vi "PM100-PM200 Utility.vi"() -> ()   [LabVIEW 2015]
uses:
  <vilib>/ptbypt/NI_PtbyPt.lvlib
  <vilib>/Utility/config.llb/NI_LVConfig.lvlib
  <vilib>/Utility/config.llb/Read Key (I32).vi
  <vilib>/Utility/config.llb/Write Key (I32).vi
  <vilib>/Utility/config.llb/Write Key (U32).vi
  StateMachine.ctl
  <vilib>/regexp/Match Regular Expression.xnode
  <vilib>/Utility/config.llb/Write Key (Double).vi
  <vilib>/Utility/config.llb/Write Key (Boolean).vi
  <vilib>/Utility/NIReport.llb/NI_ReportGenerationCore.lvlib
  <vilib>/printing/EasyPrintingControls.llb/contents.ctl
  <vilib>/printing/EasyPrintingControls.llb/orientation.ctl
  <vilib>/printing/EasyPrintingControls.llb/panel_scaling_for_page.ctl
  <vilib>/printing/EasyPrintingControls.llb/margin_values.ctl
  <vilib>/printing/EasyPrintingControls.llb/measurement_system.ctl
  <vilib>/printing/EasyPrintingControls.llb/margins.ctl
  <vilib>/printing/EasyPrintingControls.llb/printing_method.ctl
  <vilib>/printing/EasyPrintingControls.llb/color_or_monochrome.ctl
  <vilib>/printing/EasyPrintingControls.llb/printer_options.ctl
  <vilib>/printing/EasyPrintingControls.llb/page_headers.ctl
  <vilib>/printing/EasyPrintingControls.llb/page_header_content_options.ctl
  <vilib>/printing/EasyPrintingControls.llb/page_header_options.ctl
  <vilib>/printing/EasyPrintingControls.llb/layout_options.ctl
  <vilib>/printing/EasyPrintingControls.llb/report_type.ctl
  <vilib>/Utility/config.llb/Read Key (Boolean).vi
  <vilib>/Analysis/NI_AALBase.lvlib
  <vilib>/Utility/config.llb/Read Key (Double).vi
  <vilib>/Instr/_visa.llb/VISA GPIB Control REN Mode.ctl
  <vilib>/printing/EasyPrinting.llb/Easy Print VI Panel or Documentation (path).vi
panel:
  in  "att":string
  in  "Print":bool
  in  "LTM":bool caption="Long Term Measurement"
  out "Log":bool
  in  "Arm":string
  out "VI_Path":path
  in  "Button9":bool
  in  "Button10":bool
  out "Adapter":i16
  in  "Flag1":string
  in  "Flag0":string
  out "Tau":dbl
  out "Tau?":bool
  out "Temp":bool
  out "ARM":bool
  out "Stop":bool
  in  "Frame":T1
  out "Sensor?":bool
  out "SensType":i32(ring) items=["No Sensor", "Photo", "Thermo", "Pyro"]
  out "AUTO?":bool
  out "DiaIni":dbl
  out "PM100D":refnum<visa-resource-name>
  in  "Type":u16
  in  "BW":u16(ring) items=["HIGH", "LOW"]
  in  "ACC":string(combo)
  in  "Trig":dbl=5.0
  out "AOutcm²":dbl=5.0
  in  "LambdaMax":dbl=1100.0
  in  "LambdaMin":dbl=400.0
  in  "Lambda":dbl=635.0
  in  "Range Array":string[](array[string])=["AUTO", "50nA", "500nA", "5uA", "50uA", "500uA", "5mA"]
  out "Dia":dbl
  out "SlideMulti":dbl
  in  "AVG":u32=100
  out "FileRefnum":refnum<file>
  in  "File?":bool
  in  "Samples":u32=100
  out "N":u32
  out "Data":dbl
  in  "Interval":dbl=500.0
  in  "MainUnits":enum16{"W", "V", "J", "dBm", "A"}(ring)
  in  "Digits":i32=4
  in  "Sub2":enum16{"Off", "Max", "Ratio", "Area", "Second"}(ring)=enum."Max"
  in  "Sub1":enum16{"Off", "Min", "Freq", "Temp", "Res"}(ring)=enum."Min"
  in  "Button8":bool
  in  "Button7":bool
  in  "Button6":bool
  in  "Button4":bool
  in  "Button3":bool
  in  "Button2":bool
  in  "Button5":bool
  in  "Button1":bool
  out "Header":string
  out "Slide":u32(slide) scale=0.0..1000.0
  out "Sub1":string
  out "Sub2":string
  out "Readout":string
  out "FastOut":bool
  in  "FastIn":bool
  in  "Int.":i32=10 caption="Intervals" min=1 max=9999 step=1
  in  "LogCfg":string
  in  "Stat2":string
  in  "Stat1":string
  in  "Stat0":string
  out "Histogram":T2(graph)
  in  "LogData":string
  out "YT":cluster{timestamp[], dbl[]}(graph)
  out "Unit":string="Power / W"
  out "Chart_E":dbl(graph)
  out "Chart_P":dbl(graph)
  in  "Att":dbl format="%_6g"
  out "Wav":bool
  in  "Scale":bool
  out "H":dbl
  in  "Unt":string
  in  "LFP":path caption="Log-File Path"
  in  "Imp":bool
  out "N2":u32
  out "T":dbl
  in  "EMM":bool caption="Environmental Data"
  out "Hum":string caption="Rel. Humidity"
  out "Temp":string caption="Temperature"
  in  "Exp":bool
  in  "ClrGr":bool
  in  "XScaleFit":bool
  in  "YScaleRep":bool
  in  "YScaleFit":bool
  # "PM100 / PM200 Series\nOptical Power and Energy Meters"
  # "Instrument Setup"
  # "Count >"
  # "Histogram"
  # "Y-Scale"
  # "Scale Fit"
  # "Map Mode"
  # "X-Scale"
  # "Scale Fit"
  # "Scale"
  # "PM100 Utility\nVersion 4.91\n10-JUL-2013\nwww.thorlabs.com"
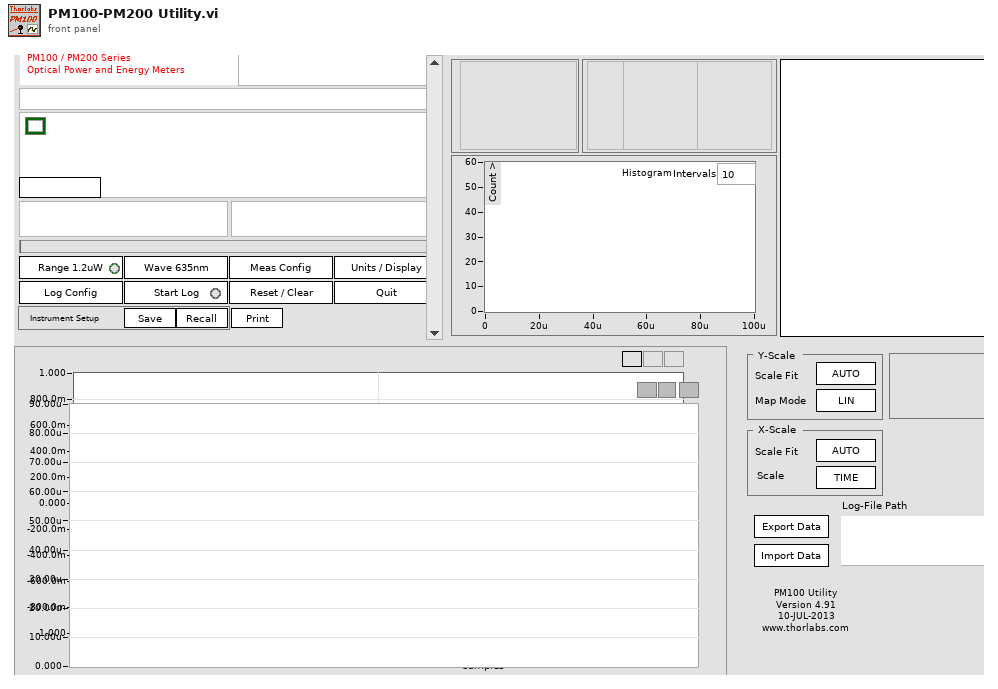
[diagram p1: front panel]
types:
  T1 = typedef "StateMachine.ctl" = enum16{"Initialize", "Load Settings", "20", "30", "40", "60", "80", "100", "120", "130", "140", "150", "160", "180", "200", "220", "240", "260", "280", "300", "320", "340", "360", "380", "400", "420", "440", "460", "480", "500", "Error", "Save Settings", "Stop"}
  T2 = cluster{"X Values":dbl[], "Histogram: h(x)":i32[]}
  T3 = enum16{"open", "replace", "create", "open or create", "replace or create", "replace or create with confirmation"}
  T4 = cluster{"X Values":i32[], "Histogram: h(x)":i32[]}
  T5 = typedef "NI_ReportGenerationCore.lvlib/layout_options.ctl" = cluster{"orientation (unchanged)":T6, "panel scaling for page (unchanged)":T7, "margins":T8, "printer options":T11, "page header options":T14}
  T6 = typedef "NI_ReportGenerationCore.lvlib/orientation.ctl" = u16
  T7 = typedef "NI_ReportGenerationCore.lvlib/panel_scaling_for_page.ctl" = u16
  T8 = typedef "NI_ReportGenerationCore.lvlib/margins.ctl" = cluster{"override VI margins (false)":bool, "margins (1.00)":T9, "measurement system (default)":T10}
  T9 = typedef "NI_ReportGenerationCore.lvlib/margin_values.ctl" = cluster{"top":dbl, "left":dbl, "right":dbl, "bottom":dbl}
  T10 = typedef "NI_ReportGenerationCore.lvlib/measurement_system.ctl" = u16
  T11 = typedef "NI_ReportGenerationCore.lvlib/printer_options.ctl" = cluster{"destination printer name (current)":string, "printing method (unchanged)":T12, "color or monochrome (unchanged)":T13}
  T12 = typedef "NI_ReportGenerationCore.lvlib/printing_method.ctl" = u16
  T13 = typedef "NI_ReportGenerationCore.lvlib/color_or_monochrome.ctl" = u16
  T14 = typedef "NI_ReportGenerationCore.lvlib/page_header_options.ctl" = cluster{"page headers (unchanged)":T15, "page header content options":T16}
  T15 = typedef "NI_ReportGenerationCore.lvlib/page_headers.ctl" = u16
  T16 = typedef "NI_ReportGenerationCore.lvlib/page_header_content_options.ctl" = cluster{"Include VI Name":bool, "Include VI Path":bool, "Include Last Modification Date":bool, "Include Date Printed":bool, "Include Page Number":bool, "Include VI Icon":bool}
  T17 = typedef "NI_LVConfig.lvlib/Config Data RefNum.ctl" = refnum<k1>
  T18 = typedef "NI_ReportGenerationCore.lvlib/report_type.ctl" = u16
  T19 = typedef "NI_ReportGenerationCore.lvlib/contents.ctl" = u16
  T20 = enum32{"invalid app kind", "Development System", "Run Time System", "Student Edition", "Embedded LabVIEW", "Evaluation", "Custom"}
  T21 = typedef "VISA GPIB Control REN Mode.ctl" = u16
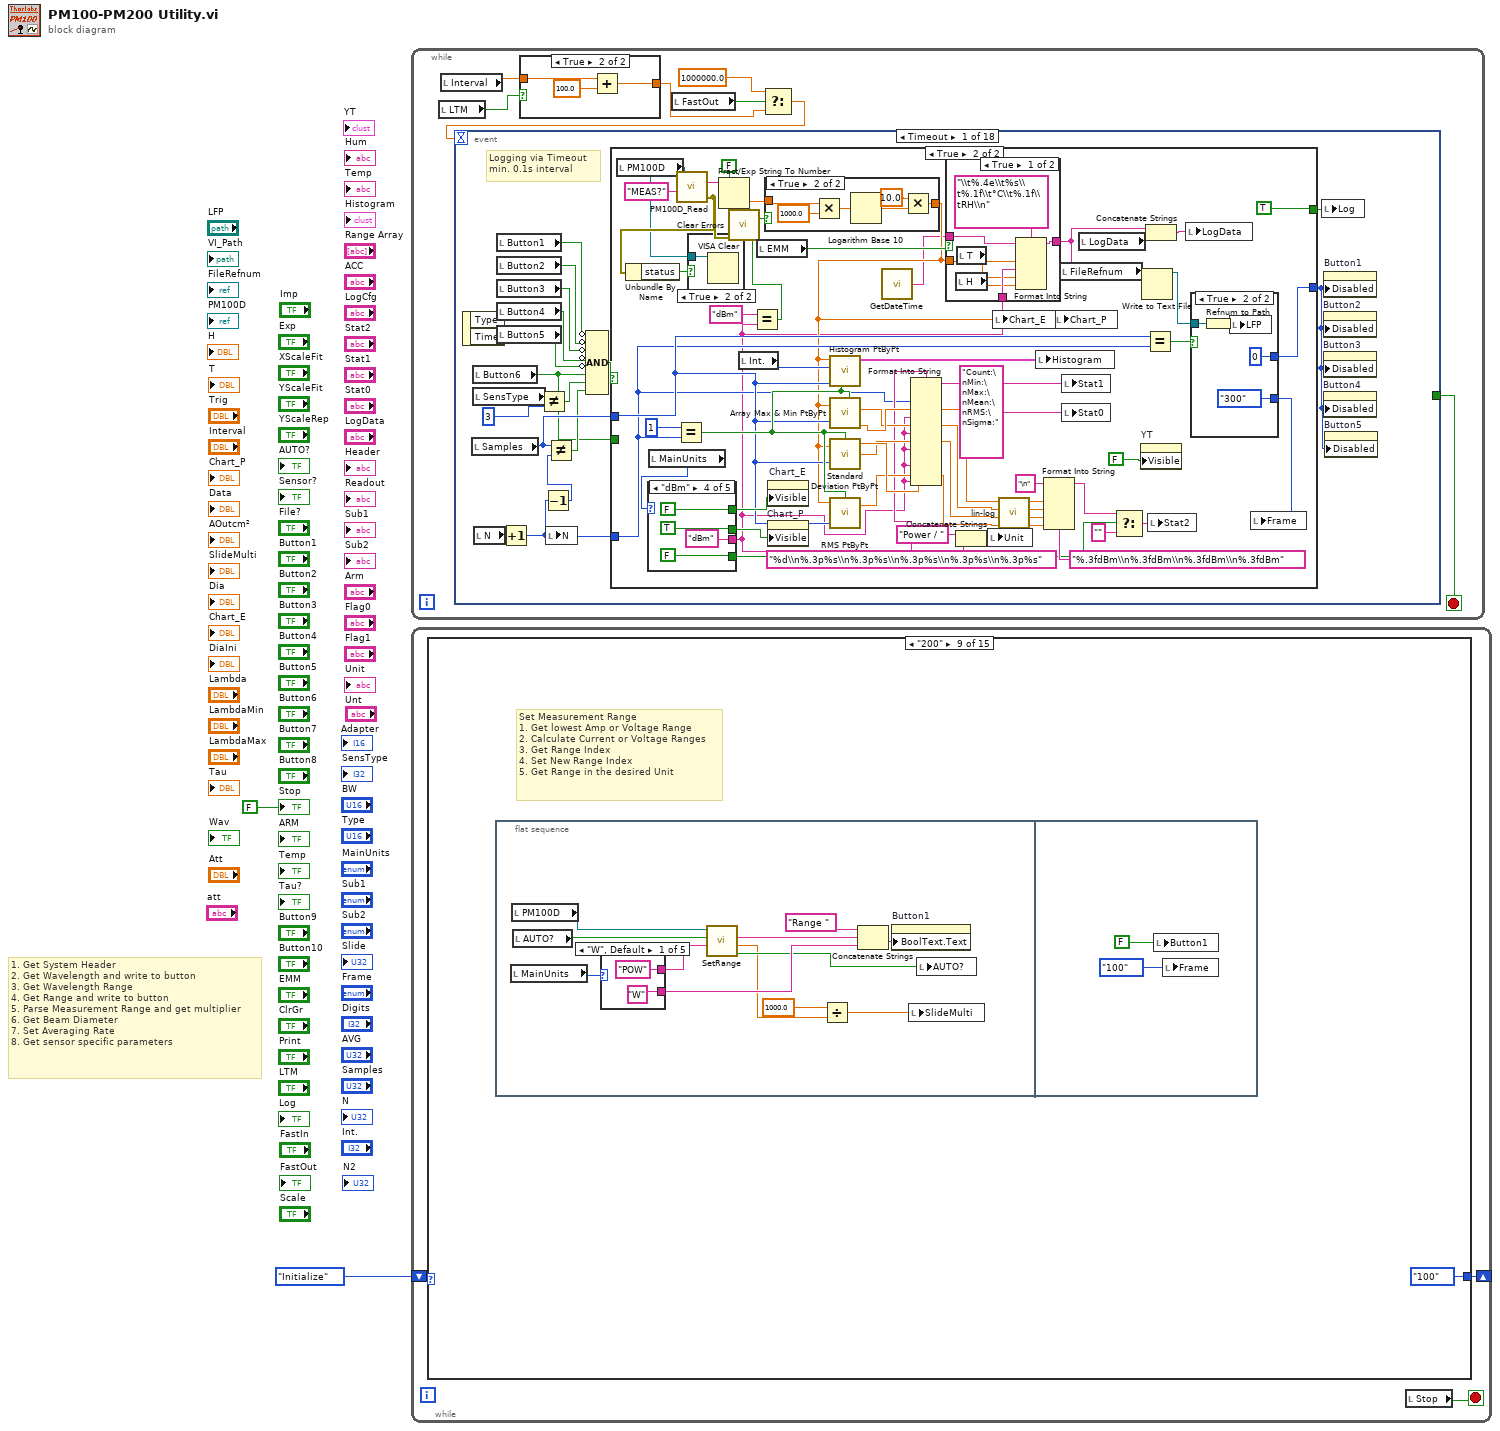
[diagram p0: block diagram]
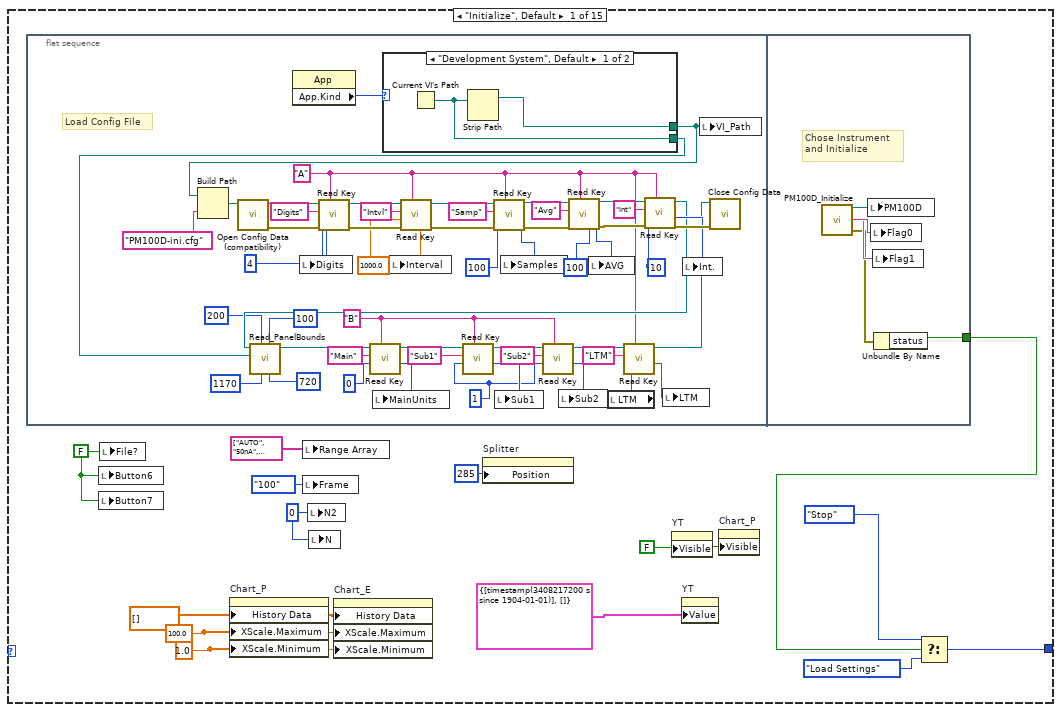
[diagram p2: hidden frame]
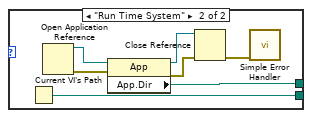
[diagram p3: hidden frame]
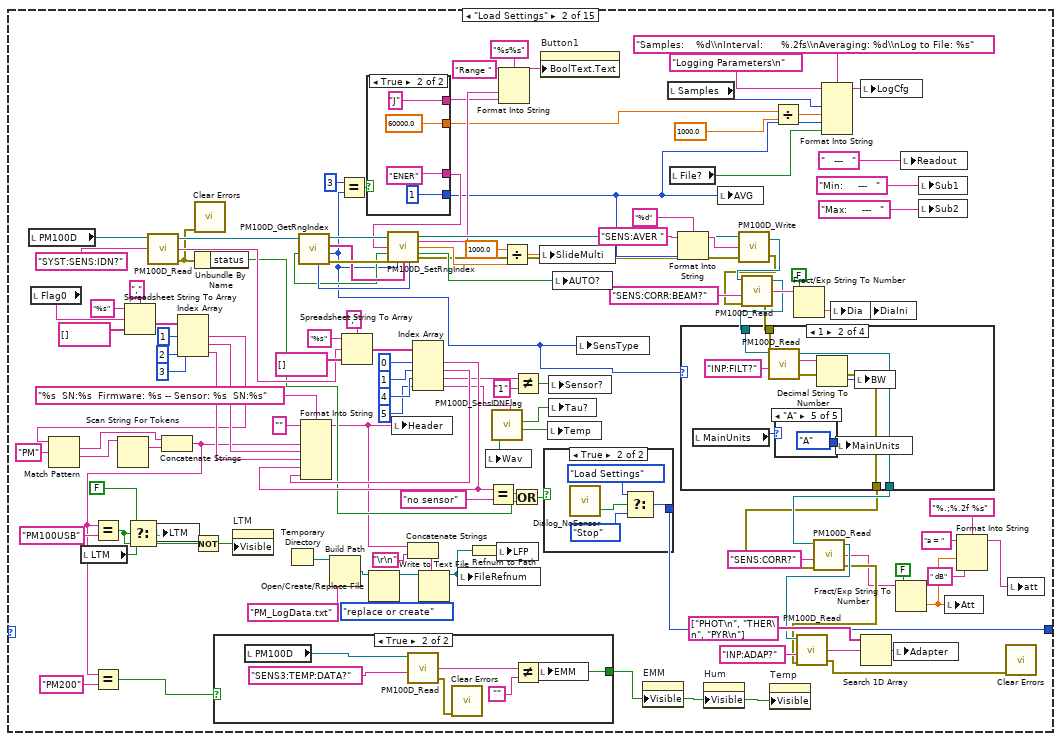
[diagram p4: hidden frame]
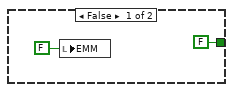
[diagram p5: hidden frame]
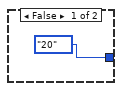
[diagram p6: hidden frame]
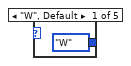
[diagram p8: hidden frame]
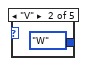
[diagram p9: hidden frame]
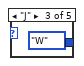
[diagram p10: hidden frame]
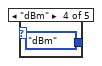
[diagram p11: hidden frame]
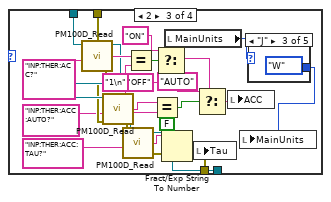
[diagram p12: hidden frame]
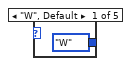
[diagram p13: hidden frame]
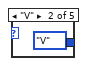
[diagram p14: hidden frame]
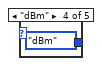
[diagram p15: hidden frame]
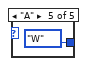
[diagram p16: hidden frame]
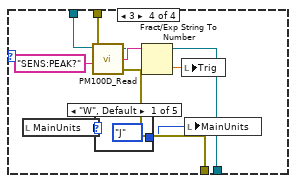
[diagram p17: hidden frame]
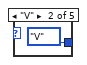
[diagram p18: hidden frame]
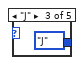
[diagram p19: hidden frame]
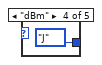
[diagram p20: hidden frame]
diagram:
  # "1. Get System Header\n2. Get Wavelength and write to button\n3. Get Wavelength Range\n4. Get Range and write to button\n5. Parse Measurement Range and get multiplier\n6. Get Beam Diameter\n7. Set Averaging Rate\n8. Get sensor specific parameters"
  n1 = while {
    stop <- w9 stop-if-true
    n2 = local read "LTM"() -> (w7:bool)
    n3 = local read "Interval"() -> (w8:dbl)
    n4 = case shown="True" w7 {
      tunnel: w8 -> [w10 w12]
      tunnel: [w10 w11] -> w4
      frame False {
      }
      frame True {
        n5 = Add(x=w12, y=100.0) -> (x+y=w11:dbl)
      }
    }
    n6 = local read "FastOut"() -> (w6:bool)
    n7 = Select(t=1000000.0, s=w6, f=w4) -> (s? t:f=w5:dbl)
    n8 = event shown="[0] Timeout" {
      selector: _ -> [_ _ _ _ _ _ _ _ _ _ _ _ _ _ _ _ _ _]
      dyn-events: _ -> [_ _ _ _ _ _ _ _ _ _ _ _ _ _ _ _ _ _]
      timeout: w5 -> [_ _ _ _ _ _ _ _ _ _ _ _ _ _ _ _ _ _]
      tunnel: [_ _ _ _ _ _ _ _ _ TRUE ("NewVal") _ _ _ _ _ _ w464 TRUE ("NewVal")] -> w9
      event Timeout {
        # "Logging via Timeout\nmin. 0.1s interval"
        n9 = event-data() -> ()  [unwired: 1 in, 2 out]
        n10 = local read "Samples"() -> (w27:u32)
        n11 = local read "Button6"() -> (w15:bool)
        n12 = local read "SensType"() -> (w25:i32)
        n13 = local read "N"() -> (w29:u32)
        n14 = local read "Button1"() -> (w16:bool)
        n15 = local read "Button2"() -> (w17:bool)
        n16 = local read "Button3"() -> (w18:bool)
        n17 = local read "Button4"() -> (w19:bool)
        n18 = local read "Button5"() -> (w20:bool)
        n19 = Increment(x=w29) -> (x+1=w26:u32)
        n20 = Not Equal?(x=w25, y=3) -> (x != y?=w22:bool)
        n21 = Decrement(x=w26) -> (x-1=w28:u32)
        n22 = Not Equal?(x=w27, y=w28) -> (x != y?=w23:bool)
        n23 = local write "N"(w26) -> ()
        n24 = Compound Arithmetic op=AND(invert w16, invert w17, invert w18, invert w19, invert w20, w15, w22, w23) -> (w30:bool)
        n25 = case shown="True" w30 {
          tunnel: w27 -> [w36 w61]
          tunnel: w26 -> [w32 w60]
          tunnel: [0 w49] -> w21
          tunnel: w15 -> [w38 _]
          tunnel: [FALSE TRUE] -> w14
          frame False {
            n26 = Equal?(x=w38, y=TRUE) -> (x = y?=w35:bool)
            n27 = Less?(x=w32, y=w36) -> (x < y?=w34:bool)
            n28 = And(x=w35, y=w34) -> (x .and. y?=w33:bool)
            n29 = case shown="True" w33 {
              frame False {
                n30 = local write "Button6"(FALSE ("Button6")) -> ()
                n31 = local write "N"(i16 0 ("N")) -> ()
              }
              frame True {
                n32 = disable-structure shown="Enabled" {
                  frame Enabled {
                    n33 = local read "N"() -> (w43:u32)
                    n34 = Decrement(x=w43) -> (x-1=w42:u32)
                    n35 = local write "N"(w42) -> ()
                  }
                  frame Disabled {
                  }
                }
              }
            }
          }
          frame True {
            n36 = local read "PM100D"() -> (w45:refnum<visa-resource-name>)
            n37 = local read "MainUnits"() -> (w90:enum16{"W", "V", "J", "dBm", "A"})
            n38 = case shown="\"dBm\"" w90 {
              tunnel: ["W" "V" "J" "dBm" "A"] -> w53
              tunnel: [w123 w126 w128 FALSE w136] -> w74
              tunnel: [FALSE w126 TRUE FALSE w136] -> w73
              tunnel: [w123 TRUE w128 TRUE TRUE] -> w72
              frame "W", Default {
                w123 = TRUE
              }
              frame "V" {
                w126 = FALSE
              }
              frame "J" {
                w128 = FALSE
              }
              frame "dBm" {
              }
              frame "A" {
                w136 = FALSE
              }
            }
            n39 = Equal?(x=i16 1, y=w60) -> (x = y?=w91:bool)
            n40 = call "PM100D_Read.vi"("Command"="MEAS?", "VISA in"=w45) -> ("error out"=w46:errorcluster, "ReadValue"=w58:string)  [unwired: 2 in, 1 out]
            n41 = Unbundle By Name(w46) -> ("status"=w44:bool)
            n42 = case shown="True" w44 {
              tunnel: w45 -> [_ w96]
              frame False {
              }
              frame True {
                n43 = VISA Clear(VISA resource name=w96) -> ()  [unwired: 1 in, 2 out]
              }
            }
            n44 = Fract/Exp String To Number(use system decimal point (T)=FALSE, string=w58) -> (number=w55:dbl)  [unwired: 2 in, 1 out]
            n45 = call <vilib>:"Clear Errors.vi"("error in (no error)"=w46) -> ()  [unwired: 5 in, 2 out]
            n46 = local read "Int."() -> (w71:i32)
            n47 = Equal?(x="dBm", y=w53) -> (x = y?=w51:bool)
            n48 = local read "EMM"() -> (w67:bool)
            n49 = case shown="True" w51 {
              tunnel: w55 -> [w97 w99]
              tunnel: [w97 w98] -> w54
              frame False {
              }
              frame True {
                n50 = Multiply(x=w99, y=1000.0) -> (x*y=w101:dbl)
                n51 = Logarithm Base 10(1:w101) -> (0:w103:dbl)
                n52 = Multiply(x=10.0, y=w103) -> (x*y=w98:dbl)
              }
            }
            n53 = property on="Chart_E" class="WFChart (strict)"("Visible"=w73) -> ()  [unwired: 2 in, 2 out]
            n54 = property on="Chart_P" class="WFChart (strict)"("Visible"=w72) -> ()  [unwired: 2 in, 2 out]
            n55 = call <vilib>:"Histogram PtByPt.vi"("initialize"=w91, "sample length"=w61, "intervals"=w71, "x"=w54) -> ("Histogram Graph"=w94:T2)  [unwired: 4 in, 3 out]
            n56 = call <vilib>:"Array Max & Min PtByPt.vi"("input data point"=w54, "sample length"=w61, "initialize"=w91) -> ("max value"=w82:dbl, "min value"=w83:dbl)  [unwired: 3 out]
            n57 = call <vilib>:"Standard Deviation PtByPt.vi"("x"=w54, "sample length"=w61, "initialize"=w91) -> ("standard deviation"=w89:dbl, "mean"=w81:dbl)  [unwired: 1 out]
            n58 = call <vilib>:"RMS PtByPt.vi"("initialize"=w91, "sample length"=w61, "x"=w54) -> ("rms value"=w80:dbl)  [unwired: 1 in, 1 out]
            n59 = call "GetDateTime.vi"() -> ("date&time"=w47:string)
            n60 = Format Into String(format string="%d\\n%.3p%s\\n%.3p%s\\n%.3p%s\\n%.3p%s\\n%.3p%s", w60, w83, w53, w82, w53, w81, w53, w80, w53, w89, w53) -> (resulting string=w93:string)  [unwired: 2 in, 1 out]
            n61 = case shown="True" w67 {
              tunnel: [w115 w120] -> w50
              tunnel: w54 -> [w114 w119]
              tunnel: w53 -> [w113 w118]
              tunnel: w47 -> [w112 w117]
              frame True {
                n62 = local read "H"() -> (w110:dbl)
                n63 = local read "T"() -> (w111:dbl)
                n64 = Format Into String(format string="\\t%.4e\\t%s\\t%.1f\\t°C\\t%.1f\\tRH\\n", initial string=w112, w114, w113, w111, w110) -> (resulting string=w115:string)  [unwired: 1 in, 1 out]
              }
              frame False {
                n65 = Format Into String(format string="\\t%.4e\\t%s\\n", initial string=w117, w119, w118) -> (resulting string=w120:string)  [unwired: 1 in, 1 out]
              }
            }
            n66 = Concatenate Strings("Power / " ("string"), w53) -> (w69:string)
            n67 = local write "Unit"(w69) -> ()
            n68 = local write "Chart_E"(w54) -> ()
            n69 = call "lin-log.vi"("W In 1"=w80, "W In 2"=w81, "W In 3"=w82, "W In 4"=w83) -> ("dBm Out 1"=w84:dbl, "dBm Out 2"=w85:dbl, "dBm Out 3"=w86:dbl, "dBm Out 4"=w87:dbl)
            n70 = local write "Histogram"(w94) -> ()
            n71 = Format Into String(format string="%.3fdBm\\n%.3fdBm\\n%.3fdBm\\n%.3fdBm", initial string="\n", w87, w86, w85, w84) -> (resulting string=w78:string)  [unwired: 1 in, 1 out]
            n72 = local write "Chart_P"(w54) -> ()
            n73 = local read "FileRefnum"() -> (w64:refnum<file>)
            n74 = local write "Stat1"(w93) -> ()
            n75 = local write "Stat0"("Count:\nMin:\nMax:\nMean:\nRMS:\nSigma:" ("Stat0")) -> ()
            n76 = local read "LogData"() -> (w65:string)
            n77 = Select(t=w78, s=w74, f="") -> (s? t:f=w77:string)
            n78 = property on="YT" class="XYGraph (strict)"("Visible"=FALSE) -> ()  [unwired: 2 in, 2 out]
            n79 = Write to Text File(file (use dialog)=w64, text=w50) -> (refnum out=w59:refnum<file>)  [unwired: 2 in, 2 out]
            n80 = Equal?(x=w61, y=w60) -> (x = y?=w62:bool)
            n81 = Concatenate Strings(w50, w65) -> (w66:string)
            n82 = local write "Stat2"(w77) -> ()
            n83 = local write "LogData"(w66) -> ()
            n84 = case shown="True" w62 {
              tunnel: [StateMachine."120" ("Frame") StateMachine."300" ("Frame")] -> w63
              tunnel: w59 -> [_ w108]
              tunnel: [2 0] -> w49
              frame False {
              }
              frame True {
                n85 = Refnum to Path(1:w108) -> (0:w107:path)
                n86 = local write "LFP"(w107) -> ()
              }
            }
            n87 = local write "Frame"(w63) -> ()
          }
        }
        n88 = local write "Log"(w14) -> ()
        n89 = property on="Button1" class="Bool (strict)"("Disabled"=w21) -> ()  [unwired: 2 in, 2 out]
        n90 = property on="Button2" class="Bool (strict)"("Disabled"=w21) -> ()  [unwired: 2 in, 2 out]
        n91 = property on="Button3" class="Bool (strict)"("Disabled"=w21) -> ()  [unwired: 2 in, 2 out]
        n92 = property on="Button4" class="Bool (strict)"("Disabled"=w21) -> ()  [unwired: 2 in, 2 out]
        n93 = property on="Button5" class="Bool (strict)"("Disabled"=w21) -> ()  [unwired: 2 in, 2 out]
      }
      event "att": Mouse Down {
        n94 = event-data() -> ()  [unwired: 1 in, 8 out]
        n95 = local write "N2"(u32 0 ("N")) -> ()
        n96 = local write "Frame"(StateMachine."240" ("Frame")) -> ()
      }
      event "Button1": Value Change {
        # "Set Range - goto Frame 200"
        n97 = event-data() -> ("NewVal"=w143:bool)  [unwired: 1 in, 5 out]
        n98 = Equal?(x=w143, y=TRUE) -> (x = y?=w141:bool)
        n99 = case shown="True" w141 {
          frame False {
          }
          frame True {
            n100 = local write "Frame"(StateMachine."200" ("Frame")) -> ()
          }
        }
        n101 = local write "N2"(u32 0 ("N2")) -> ()
      }
      event "Button2": Value Change {
        # "Set Wavelength - goto Frame 220"
        n102 = event-data() -> ("NewVal"=w148:bool)  [unwired: 1 in, 5 out]
        n103 = Equal?(x=w148, y=TRUE) -> (x = y?=w146:bool)
        n104 = case shown="True" w146 {
          frame False {
          }
          frame True {
            n105 = local write "Frame"(StateMachine."220" ("Frame")) -> ()
          }
        }
        n106 = local write "N2"(u32 0 ("N2")) -> ()
      }
      event "Button3": Value Change {
        # "Set Measuremnt Configuration - goto Frame 240"
        n107 = event-data() -> ("NewVal"=w153:bool)  [unwired: 1 in, 5 out]
        n108 = Equal?(x=w153, y=TRUE) -> (x = y?=w151:bool)
        n109 = case shown="True" w151 {
          frame False {
          }
          frame True {
            n110 = local write "Frame"(StateMachine."240" ("Frame")) -> ()
          }
        }
        n111 = local write "N2"(u32 0 ("N2")) -> ()
      }
      event "Button4": Value Change {
        # "Set Units - goto Frame 260"
        n112 = event-data() -> ("NewVal"=w158:bool)  [unwired: 1 in, 5 out]
        n113 = Equal?(x=w158, y=TRUE) -> (x = y?=w156:bool)
        n114 = case shown="True" w156 {
          frame False {
          }
          frame True {
            n115 = local write "Frame"(StateMachine."260" ("Frame")) -> ()
          }
        }
        n116 = local write "N2"(u32 0 ("N2")) -> ()
      }
      event "Button5": Value Change {
        # "Set Logging Parameters Goto 280"
        n117 = event-data() -> ("NewVal"=w163:bool)  [unwired: 1 in, 5 out]
        n118 = Equal?(x=w163, y=TRUE) -> (x = y?=w161:bool)
        n119 = case shown="True" w161 {
          frame False {
          }
          frame True {
            n120 = local write "Frame"(StateMachine."280" ("Frame")) -> ()
          }
        }
        n121 = local write "N2"(u32 0 ("N2")) -> ()
      }
      event "Button6": Value Change {
        # "Start/Stop"
        n122 = event-data() -> ()  [unwired: 1 in, 6 out]
        n123 = local read "Button6"() -> (w167:bool)
        n124 = Equal?(x=w167, y=FALSE) -> (x = y?=w165:bool)
        n125 = case shown="True" w165 {
          frame False {
          }
          frame True {
            n126 = local write "Frame"(StateMachine."300" ("Frame")) -> ()
          }
        }
      }
      event "Button7": Value Change {
        w182 = 1.0 ("X Scale.Range:Minimum")
        w183 = 100.0 ("X Scale.Range:Maximum")
        w181 = i16 0 ("N")
        w187 = dbl[] [] ("History Data")
        w172 = ""
        # "Reset/Clear"
        n127 = event-data() -> ()  [unwired: 1 in, 6 out]
        n128 = Temporary Directory() -> (w169:path)
        n129 = local write "N"(w181) -> ()
        n130 = local write "LogData"(w172) -> ()
        n131 = Build Path(base path=w169, name or relative path="PM_LogData.txt") -> (appended path=w179:path)
        n132 = property on="Chart_P" class="WFChart (strict)"("History Data"=w187, "XScale.Maximum"=w183, "XScale.Minimum"=w182) -> ()  [unwired: 2 in, 2 out]
        n133 = local write "Histogram"(T4 {"X Values"=[], "Histogram: h(x)"=[]} ("Histogram Graph")) -> ()
        n134 = local write "N2"(w181) -> ()
        n135 = local write "Stat2"(w172) -> ()
        n136 = local read "Header"() -> (w175:string)
        n137 = Open/Create/Replace File(file path (use dialog)=w179, operation (0:open)=T3."replace or create") -> (refnum out=w177:refnum<file>)  [unwired: 4 in, 2 out]
        n138 = local write "Stat1"(w172) -> ()
        n139 = property on="Chart_E" class="WFChart (strict)"("History Data"=w187, "XScale.Maximum"=w183, "XScale.Minimum"=w182) -> ()  [unwired: 2 in, 2 out]
        n140 = Concatenate Strings(w175, "\r\n") -> (w173:string)
        n141 = Write to Text File(file (use dialog)=w177, text=w173) -> (refnum out=w171:refnum<file>, error out=w174:errorcluster)  [unwired: 2 in, 1 out]
        n142 = local write "Frame"(StateMachine."100" ("Frame")) -> ()
        n143 = local read "File?"() -> (w170:bool)
        n144 = local write "Readout"("   ---   " ("Readout")) -> ()
        n145 = local write "Sub1"("Min:     ---   " ("Sub1")) -> ()
        n146 = local write "Sub2"("Max:     ---   " ("Sub2")) -> ()
        n147 = call <vilib>:"Clear Errors.vi"("error in (no error)"=w174) -> ()  [unwired: 5 in, 2 out]
        n148 = case shown="False" w170 {
          tunnel: w171 -> [w191 _]
          frame False {
            n149 = local write "FileRefnum"(w191) -> ()
            n150 = Refnum to Path(1:w191) -> (0:w190:path)
            n151 = local write "LFP"(w190) -> ()
          }
          frame True {
          }
        }
      }
      event "Button8": Value Change {
        # "Quit"
        n152 = event-data() -> ("NewVal"=w195:bool)  [unwired: 1 in, 5 out]
        n153 = Equal?(x=w195, y=TRUE) -> (x = y?=w194:bool)
        n154 = case shown="True" w194 {
          selector: w194 -> [_ w199]
          frame False {
          }
          frame True {
            n155 = flat-sequence {
              tunnel: w199 -> [w235]
              tunnel: [FALSE ("Button8")] -> w198
              tunnel: [TRUE] -> w197
              frame #0 {
                w213 = "B" ("section")
                w202 = "A" ("section")
                n156 = Current VI's Path() -> (path=w219:path)
                n157 = local write "Stop"(w235) -> ()
                n158 = local read "VI_Path"() -> (w206:path)
                n159 = local read "PM100D"() -> (w237:refnum<visa-resource-name>)
                n160 = local write "Frame"(StateMachine."Stop" ("Frame")) -> ()
                n161 = call "PM100D_Close.vi"("VISA resource name"=w237) -> ()  [unwired: 3 in]
                n162 = Build Path(base path=w206, name or relative path="PM100D-ini.cfg") -> (appended path=w234:path)
                n163 = local read "SensType"() -> (w222:i32)
                n164 = local read "Digits"() -> (w231:i32)
                n165 = call <vilib>:"Open Config Data (compatibility).vi"("configuration file path"=w234) -> ("refnum"=w226:T17)  [unwired: 8 in, 2 out]
                n166 = Equal?(x=w222, y=3) -> (x = y?=w220:bool)
                n167 = local read "MainUnits"() -> (w209:enum16{"W", "V", "J", "dBm", "A"})
                n168 = call-poly <vilib>:"Write Key.vi"("section"=w202, "value"=w231, "key"="Digits", "refnum"=w226) -> ("refnum out"=w228:T17)  [unwired: 5 in, 2 out]
                n169 = case shown="False" w220 {
                  tunnel: [w240 w247] -> w230
                  tunnel: w228 -> [w245 w247]
                  tunnel: w202 -> [w243 _]
                  tunnel: w202 -> [w238 _]
                  frame False {
                    n170 = local read "Interval"() -> (w246:dbl)
                    n171 = call-poly <vilib>:"Write Key.vi"("section"=w243, "value"=w246, "key"="Intvl", "refnum"=w245) -> ("refnum out"=w239:T17)  [unwired: 5 in, 2 out]
                    n172 = local read "AVG"() -> (w242:u32)
                    n173 = call-poly <vilib>:"Write Key.vi"("section"=w238, "value"=w242, "key"="Avg", "refnum"=w239) -> ("refnum out"=w240:T17)  [unwired: 5 in, 2 out]
                  }
                  frame True {
                  }
                }
                n174 = local read "Sub1"() -> (w207:enum16{"Off", "Min", "Freq", "Temp", "Res"})
                n175 = local read "Sub2"() -> (w208:enum16{"Off", "Max", "Ratio", "Area", "Second"})
                n176 = local read "Samples"() -> (w232:u32)
                n177 = call-poly <vilib>:"Write Key.vi"("section"=w202, "value"=w232, "key"="Samp", "refnum"=w230) -> ("refnum out"=w217:T17)  [unwired: 5 in, 2 out]
                n178 = local read "LTM"() -> (w201:bool)
                n179 = local read "Int."() -> (w224:i32)
                n180 = call-poly <vilib>:"Write Key.vi"("section"=w202, "value"=w224, "key"="Int", "refnum"=w217) -> ("refnum out"=w218:T17)  [unwired: 5 in, 2 out]
                n181 = call "Write_PanelBounds.vi"("refnum in"=w218, "path"=w219) -> ("refnum out"=w216:T17)
                n182 = call-poly <vilib>:"Write Key.vi"("section"=w213, "value"=w209, "key"="Main", "refnum"=w216) -> ("refnum out"=w215:T17)  [unwired: 5 in, 2 out]
                n183 = call-poly <vilib>:"Write Key.vi"("section"=w213, "value"=w207, "key"="Sub1", "refnum"=w215) -> ("refnum out"=w214:T17)  [unwired: 5 in, 2 out]
                n184 = call-poly <vilib>:"Write Key.vi"("section"=w213, "value"=w208, "key"="Sub2", "refnum"=w214) -> ("refnum out"=w204:T17)  [unwired: 5 in, 2 out]
                n185 = call-poly <vilib>:"Write Key.vi"("section"=w202, "value"=w201, "key"="LTM", "refnum"=w204) -> ("refnum out"=w203:T17)  [unwired: 5 in, 2 out]
                n186 = call <vilib>:"Close Config Data.vi"("refnum"=w203) -> ()  [unwired: 9 in, 2 out]
              }
            }
            n187 = local write "Button8"(w198) -> ()
            n188 = Quit LabVIEW(quit? (T)=w197) -> ()
          }
        }
        n189 = local write "N2"(u32 0 ("N2")) -> ()
      }
      event "Button9": Value Change {
        # "Recall Instrument Setup"
        n190 = event-data() -> ()  [unwired: 1 in, 6 out]
        n191 = local read "VI_Path"() -> (w249:path)
        n192 = call "File Dialog2"("start path"=w249, "default name"="PM100 Setup_1", "pattern (all files)"="*.txt", "pattern label"="Textfile") -> ("selected path"=w256:path, "cancelled"=w252:bool, "error out"=w254:errorcluster)  [unwired: 8 in, 1 out]
        n193 = local write "N2"(u32 0 ("N2")) -> ()
        n194 = Open/Create/Replace File(file path (use dialog)=w256, error in=w254, operation (0:open)=T3."open") -> (refnum out=w251:refnum<file>, error out=w257:errorcluster)  [unwired: 3 in, 1 out]
        n195 = call <vilib>:"Clear Errors.vi"("error in (no error)"=w257) -> ()  [unwired: 5 in, 2 out]
        n196 = case shown="False" w252 {
          tunnel: w251 -> [w322 _]
          frame False {
            w279 = 0 ("default value 8")
            n197 = local read "PM100D"() -> (w271:refnum<visa-resource-name>)
            n198 = local read "Lambda"() -> (w320:dbl)
            n199 = local read "Adapter"() -> (w281:i16)
            n200 = local read "Tau"() -> (w319:dbl)
            n201 = local read "Dia"() -> (w318:dbl)
            n202 = local read "BW"() -> (w302:u16)
            n203 = local read "SensType"() -> (w278:i32)
            n204 = local read "Sensor?"() -> (w303:bool)
            n205 = local read "MainUnits"() -> (w268:enum16{"W", "V", "J", "dBm", "A"})
            n206 = Scan From String("%d %f %f %f %d %d %d %d" ("format string"), w322, default 1=1 ("default value 1"), default 2=w320, default 3=w319, default 4=w318, default 5=w281, default 6=w302, default 7=w279, default 8=w279) -> (w285:refnum<file>, w288:errorcluster, output 1=w287:i32, output 2=w306:dbl, output 3=w312:dbl, output 4=w317:dbl, output 5=w282:i16, output 6=w299:u16, output 7=w273:i32, output 8=w275:i32)  [unwired: 1 in]
            n207 = Number To Boolean Array(number=w275) -> (Boolean array=w277:bool[])
            n208 = Index Array(array=w277, index=0) -> (element=w274:bool)
            n209 = case shown="\"dBm\"" w268 {
              tunnel: ["POW" "VOLT" "ENER" "POW" "CURR"] -> w267
              tunnel: ["W" "V" "J" "W" "A"] -> w260
              frame "W", Default {
              }
              frame "V" {
              }
              frame "J" {
              }
              frame "dBm" {
              }
              frame "A" {
              }
            }
            n210 = Not Equal?(x=w282, y=w281) -> (x != y?=w280:bool)
            n211 = local write "Lambda"(w306) -> ()
            n212 = local write "Adapter"(w282) -> ()
            n213 = call <vilib>:"Clear Errors.vi"("error in (no error)"=w288) -> ()  [unwired: 5 in, 2 out]
            n214 = local write "Tau"(w312) -> ()
            n215 = local write "Dia"(w317) -> ()
            n216 = call "PM100D_Ranging.vi"("VISA in"=w271, "Index"=w273, "AUTO"=w274, "Unit"=w267) -> ("AUTO?"=w266:bool, "VISA out"=w270:refnum<visa-resource-name>, "RANG_Val"=w265:dbl, "RANG_lbl"=w259:string, "error out"=w269:errorcluster)  [unwired: 4 in, 3 out]
            n217 = case shown="0" w287 {
              tunnel: [" ON" ("ACCOut") " OFF" ("ACCOut") ":AUTO ON" ("ACCOut")] -> w307
              tunnel: ["ON" ("ACCOut") "OFF" ("ACCOut") "AUTO" ("ACCOut")] -> w286
              frame 0 {
              }
              frame 2 {
              }
              frame 1, Default {
              }
            }
            n218 = local write "BW"(w299) -> ()
            n219 = Close File(refnum=w285) -> ()  [unwired: 1 in, 2 out]
            n220 = local write "ACC"(w286) -> ()
            n221 = Format Into String(format string="%.;%f", initial string="INP:THER:ACC:TAU ", w312) -> (resulting string=w313:string)  [unwired: 1 in, 1 out]
            n222 = Format Into String(format string="%.;%f", initial string="SENS:CORR:BEAM ", w317) -> (resulting string=w316:string)  [unwired: 1 in, 1 out]
            n223 = local write "AUTO?"(w266) -> ()
            n224 = Format Into String(format string="INP:THER:ACC%s", w307) -> (resulting string=w308:string)  [unwired: 2 in, 1 out]
            n225 = call "PM100D_Write.vi"("error in (no error)"=w269, "Command"=w308, "VISA in"=w270) -> ("error out"=w293:errorcluster, "VISA out"=w298:refnum<visa-resource-name>)
            n226 = call "PM100D_Write.vi"("error in (no error)"=w293, "Command"=w313, "VISA in"=w298) -> ("error out"=w292:errorcluster, "VISA out"=w297:refnum<visa-resource-name>)
            n227 = call "PM100D_Write.vi"("error in (no error)"=w292, "Command"=w316, "VISA in"=w297) -> ("error out"=w291:errorcluster, "VISA out"=w296:refnum<visa-resource-name>)
            n228 = case shown="True" w280 {
              tunnel: w296 -> [w334 w339]
              tunnel: [w334 w338] -> w295
              tunnel: w291 -> [w333 w337]
              tunnel: [w333 w336] -> w289
              tunnel: w282 -> [_ w335]
              frame False {
              }
              frame True {
                n229 = case shown="0, Default" w335 {
                  tunnel: ["INP:ADAP PHOT" "INP:ADAP THER" "INP:ADAP PYR"] -> w340
                  frame 0, Default {
                  }
                  frame 1 {
                  }
                  frame 2 {
                  }
                }
                n230 = call "PM100D_Write.vi"("error in (no error)"=w337, "Command"=w340, "VISA in"=w339) -> ("error out"=w336:errorcluster, "VISA out"=w338:refnum<visa-resource-name>)
              }
            }
            n231 = case shown="True" w303 {
              tunnel: w306 -> [w346 _]
              tunnel: [w345 w352] -> w304
              tunnel: [w344 w351] -> w305
              tunnel: w278 -> [_ w354]
              tunnel: w306 -> [_ w353]
              frame True {
                n232 = Format Into String(format string="%dnm", initial string="Wave ", w346) -> (resulting string=w345:string)  [unwired: 1 in, 1 out]
                n233 = Format Into String(format string="%d", initial string="SENS:CORR:WAV " ("Command"), w346) -> (resulting string=w344:string)  [unwired: 1 in, 1 out]
              }
              frame False {
                n234 = case shown="1" w354 {
                  tunnel: [w359 "" ("initial string") "" ("initial string") "" ("initial string")] -> w358
                  tunnel: [w359 "%.;%_3pA/W" ("format string") "%.;%_3pV/W" ("format string") "%.;%_3pV/J" ("format string")] -> w357
                  tunnel: [w359 "SENS:CORR:POW " ("Command") "SENS:CORR:POW:THER " ("Command") "SENS:CORR:ENER " ("Command")] -> w356
                  tunnel: [w359 "%.;%.6e" ("format string") "%.;%.6e" ("format string") "%.;%.6e" ("format string")] -> w355
                  frame 0, Default {
                    w359 = "" ("format string")
                  }
                  frame 1 {
                  }
                  frame 2 {
                  }
                  frame 3 {
                  }
                }
                n235 = Format Into String(format string=w357, initial string=w358, w353) -> (resulting string=w352:string)  [unwired: 1 in, 1 out]
                n236 = Format Into String(format string=w355, initial string=w356, w353) -> (resulting string=w351:string)  [unwired: 1 in, 1 out]
              }
            }
            n237 = Divide(x=1000.0, y=w265) -> (x/y=w263:dbl)
            n238 = local write "SlideMulti"(w263) -> ()
            n239 = Format Into String(format string="INP:FILT %d", w299) -> (resulting string=w301:string)  [unwired: 2 in, 1 out]
            n240 = Concatenate Strings("Range " ("string"), w259, w260) -> (w262:string)
            n241 = property on="Button1" class="Bool (strict)"("BoolText.Text"=w262) -> ()  [unwired: 2 in, 2 out]
            n242 = property on="Button2" class="Bool (strict)"("BoolText.Text"=w304) -> ()  [unwired: 2 in, 2 out]
            n243 = call "PM100D_Write.vi"("error in (no error)"=w289, "Command"=w305, "VISA in"=w295) -> ("error out"=w290:errorcluster, "VISA out"=w294:refnum<visa-resource-name>)
            n244 = call "PM100D_Write.vi"("error in (no error)"=w290, "Command"=w301, "VISA in"=w294) -> ("error out"=w272:errorcluster)  [unwired: 1 out]
            n245 = local write "Button9"(FALSE ("Load")) -> ()
            n246 = call <vilib>:"Clear Errors.vi"("error in (no error)"=w272) -> ()  [unwired: 5 in, 2 out]
          }
          frame True {
          }
        }
      }
      event "Button10": Value Change {
        # "Save Instrument Setup"
        n247 = event-data() -> ()  [unwired: 1 in, 6 out]
        n248 = local read "VI_Path"() -> (w380:path)
        n249 = call "File Dialog"("start path"=w380, "default name"="PM100 Setup_1", "pattern (all files)"="*.txt", "pattern label"="Textfile") -> ("selected path"=w387:path, "cancelled"=w383:bool, "error out"=w384:errorcluster)  [unwired: 8 in, 1 out]
        n250 = Open/Create/Replace File(file path (use dialog)=w387, error in=w384, operation (0:open)=T3."replace or create") -> (refnum out=w390:refnum<file>, error out=w388:errorcluster)  [unwired: 3 in, 1 out]
        n251 = local read "PM100D"() -> (w379:refnum<visa-resource-name>)
        n252 = call <vilib>:"Clear Errors.vi"("error in (no error)"=w388) -> ()  [unwired: 5 in, 2 out]
        n253 = case shown="False" w383 {
          tunnel: w390 -> [w406 _]
          tunnel: w379 -> [w395 _]
          frame False {
            n254 = call "PM100D_GetRngIndex.vi"("VISA in"=w395) -> ("error out"=w391:errorcluster, "IndexOut"=w394:i32, "AutoOut"=w393:bool)  [unwired: 5 in, 3 out]
            n255 = call <vilib>:"Clear Errors.vi"("error in (no error)"=w391) -> ()  [unwired: 5 in, 2 out]
            n256 = local read "ACC"() -> (w397:string)
            n257 = local read "Lambda"() -> (w405:dbl)
            n258 = local read "Adapter"() -> (w402:i16)
            n259 = local read "Tau"() -> (w404:dbl)
            n260 = local read "Dia"() -> (w403:dbl)
            n261 = local read "BW"() -> (w399:u16)
            n262 = case shown="\" OFF\"" w397 {
              tunnel: [0 0 1 1 2 2] -> w396
              frame "ON", Default {
              }
              frame " ON" {
              }
              frame "AUTO" {
              }
              frame ":AUTO ON" {
              }
              frame "OFF" {
              }
              frame " OFF" {
              }
            }
            n263 = Boolean To (0,1)(Boolean=w393) -> (0, 1=w392:i16)
            n264 = Format Into String(format string="%d %f %f %f %d %d %d %d", initial string=w406, w396, w405, w404, w403, w402, w399, w394, w392) -> (resulting string=w400:refnum<file>, error out=w398:errorcluster)  [unwired: 1 in]
            n265 = call <vilib>:"Clear Errors.vi"("error in (no error)"=w398) -> ()  [unwired: 5 in, 2 out]
            n266 = Close File(refnum=w400) -> ()  [unwired: 1 in, 2 out]
          }
          frame True {
          }
        }
        n267 = local write "N2"(u32 0 ("N2")) -> ()
        n268 = local write "Button10"(FALSE ("Save")) -> ()
      }
      event "ClrGr": Value Change {
        n269 = event-data() -> ()  [unwired: 1 in, 6 out]
        n270 = flat-sequence {
          frame #0 {
            w414 = 1.0 ("X Scale.Range:Minimum")
            w415 = 100.0 ("X Scale.Range:Maximum")
            w416 = dbl[] [] ("History Data")
            n271 = disable-structure shown="Disabled" {
              frame Disabled {
                w422 = ""
                n272 = local write "LogData"(w422) -> ()
                n273 = local write "Histogram"(T4 {"X Values"=[], "Histogram: h(x)"=[]} ("Histogram Graph")) -> ()
                n274 = local write "Stat2"(w422) -> ()
                n275 = local write "Stat1"(w422) -> ()
                n276 = local write "N"(i16 0 ("N")) -> ()
                n277 = local write "Readout"("   ---   " ("Readout")) -> ()
                n278 = local write "Sub1"("Min:     ---   " ("Sub1")) -> ()
                n279 = local write "Sub2"("Max:     ---   " ("Sub2")) -> ()
              }
              frame Enabled {
              }
            }
            n280 = property on="Chart_P" class="WFChart (strict)"("History Data"=w416, "XScale.Maximum"=w415, "XScale.Minimum"=w414) -> ()  [unwired: 2 in, 2 out]
            n281 = property on="Chart_E" class="WFChart (strict)"("History Data"=w416, "XScale.Maximum"=w415, "XScale.Minimum"=w414) -> ()  [unwired: 2 in, 2 out]
            n282 = local write "Frame"(StateMachine."100" ("Frame")) -> ()
            n283 = property on="YT" class="XYGraph (strict)"("Value"=cluster{timestamp[], dbl[]} {[timestamp(3408217200 s since 1904-01-01)], []} ("YT")) -> ()  [unwired: 2 in, 2 out]
          }
          frame #1 {
            n284 = local write "ClrGr"(FALSE ("ClrGr")) -> ()
          }
        }
      }
      event "Imp": Value Change {
        # "Import Logging Data"
        n285 = event-data() -> ("NewVal"=w426:bool)  [unwired: 1 in, 5 out]
        n286 = Equal?(x=w426, y=TRUE) -> (x = y?=w425:bool)
        n287 = case shown="True" w425 {
          frame False {
          }
          frame True {
            n288 = local read "LFP"() -> (w431:path)
            n289 = Strip Path(path=w431) -> (name=w430:string)  [unwired: 1 out]
            n290 = call "File Dialog4"("start path"=w431, "default name"=w430) -> ("selected path"=w433:path, "cancelled"=w434:bool, "error out"=w429:errorcluster)  [unwired: 10 in, 1 out]
            n291 = call <vilib>:"Clear Errors.vi"("error in (no error)"=w429) -> ()  [unwired: 5 in, 2 out]
            n292 = case shown="False" w434 {
              tunnel: [w436 w438] -> w432
              tunnel: w433 -> [w436 _]
              tunnel: [StateMachine."300" ("Frame") StateMachine."300" ("Frame")] -> w428
              frame False {
              }
              frame True {
                n293 = local read "LFP"() -> (w438:path)
              }
            }
            n294 = local write "LFP"(w432) -> ()
            n295 = local write "Frame"(w428) -> ()
          }
        }
      }
      event "Exp": Value Change {
        # "Export\nData"
        n296 = event-data() -> ()  [unwired: 1 in, 6 out]
        n297 = flat-sequence {
          frame #0 {
            n298 = call <vilib>:"Dflt Data Dir.vi"() -> ("App:Default Data Directory"=w440:path)
            n299 = call "File Dialog3"("start path"=w440, "prompt"="PM100 LogData" ("default name"), "default name"="PM_LogData", "pattern (all files)"="*.txt", "pattern label"="Textfile") -> ("selected path"=w439:path, "cancelled"=w446:bool, "error out"=w447:errorcluster)  [unwired: 7 in, 1 out]
            n300 = local read "LogData"() -> (w444:string)
            n301 = Open/Create/Replace File(file path (use dialog)=w439, error in=w447, operation (0:open)=T3."replace or create with confirmation") -> (refnum out=w445:refnum<file>, error out=w450:errorcluster)  [unwired: 3 in, 1 out]
            n302 = local write "LFP"(w439) -> ()
            n303 = case shown="False" w446 {
              tunnel: w444 -> [w452 _]
              tunnel: w445 -> [w455 _]
              frame False {
                n304 = Format Into String(format string="%s", initial string=w455, w452) -> (resulting string=w454:refnum<file>)  [unwired: 1 in, 1 out]
                n305 = Close File(refnum=w454) -> ()  [unwired: 1 in, 2 out]
              }
              frame True {
              }
            }
            n306 = call <vilib>:"Clear Errors.vi"("error in (no error)"=w450) -> ()  [unwired: 5 in, 2 out]
            n307 = local write "N2"(u32 0 ("N2")) -> ()
          }
          frame #1 {
            n308 = local write "Exp"(FALSE ("Exp")) -> ()
          }
        }
      }
      event "Print": Value Change {
        w458 = T18 0 items=["Quick Print", "Standard Report", "HTML"] ("report type (Quick Print)")
        w460 = T19 0 items=["Complete front panel", "Visible portion of front panel", "Icon, description, panel and diagram", "Documentation: Using the panel", "Documentation: Using as a subVI", "Documentation: Complete", "Documentation: Custom"] ("contents (complete front panel)")
        # "Print Front-Panel"
        n309 = event-data() -> ()  [unwired: 1 in, 6 out]
        n310 = local write "Print"(FALSE ("Print")) -> ()
        n311 = local write "N2"(u32 0 ("N2")) -> ()
        n312 = Current VI's Path() -> (path=w461:path)
        n313 = call-poly <vilib>:"Easy Print VI Panel or Documentation.vi"("layout options"=T5 {"orientation (unchanged)"=0, "panel scaling for page (unchanged)"=0, "margins"={"override VI margins (false)"=FALSE, "margins (1.00)"={"top"=1.0, "left"=1.0, "right"=1.0, "bottom"=1.0}, "measurement system (default)"=0}, "printer options"={"destination printer name (current)"="", "printing method (unchanged)"=0, "color or monochrome (unchanged)"=0}, "page header options"={"page headers (unchanged)"=0, "page header content options"={"Include VI Name"=TRUE, "Include VI Path"=FALSE, "Include Last Modification Date"=FALSE, "Include Date Printed"=TRUE, "Include Page Number"=FALSE, "Include VI Icon"=FALSE}}}, "report type (Quick Print)"=w458, "contents (complete front panel)"=w460, "VI path"=w461) -> ()  [unwired: 6 in, 2 out]
      }
      event "Stop": Value Change {
        n314 = event-data() -> ("NewVal"=w464:bool)  [unwired: 1 in, 5 out]
        n315 = local write "Frame"(StateMachine."Stop" ("Frame")) -> ()
      }
      event Panel Close {
        n316 = event-data() -> ()  [unwired: 1 in, 3 out]
        n317 = case shown="True" TRUE ("y") {
          selector: TRUE ("y") -> [_ w469]
          frame False {
          }
          frame True {
            n318 = flat-sequence {
              tunnel: w469 -> [w505]
              tunnel: [FALSE ("Button8")] -> w468
              tunnel: [TRUE] -> w467
              frame #0 {
                w483 = "B" ("section")
                w472 = "A" ("section")
                n319 = Current VI's Path() -> (path=w489:path)
                n320 = local write "Stop"(w505) -> ()
                n321 = local read "VI_Path"() -> (w476:path)
                n322 = local read "PM100D"() -> (w507:refnum<visa-resource-name>)
                n323 = local write "Frame"(StateMachine."Stop" ("Frame")) -> ()
                n324 = call "PM100D_Close.vi"("VISA resource name"=w507) -> ()  [unwired: 3 in]
                n325 = Build Path(base path=w476, name or relative path="PM100D-ini.cfg") -> (appended path=w504:path)
                n326 = local read "SensType"() -> (w492:i32)
                n327 = local read "Digits"() -> (w501:i32)
                n328 = call <vilib>:"Open Config Data (compatibility).vi"("configuration file path"=w504) -> ("refnum"=w496:T17)  [unwired: 8 in, 2 out]
                n329 = Equal?(x=w492, y=3) -> (x = y?=w490:bool)
                n330 = local read "MainUnits"() -> (w479:enum16{"W", "V", "J", "dBm", "A"})
                n331 = call-poly <vilib>:"Write Key.vi"("section"=w472, "value"=w501, "key"="Digits", "refnum"=w496) -> ("refnum out"=w498:T17)  [unwired: 5 in, 2 out]
                n332 = case shown="False" w490 {
                  tunnel: [w510 w517] -> w500
                  tunnel: w498 -> [w515 w517]
                  tunnel: w472 -> [w513 _]
                  tunnel: w472 -> [w508 _]
                  frame False {
                    n333 = local read "Interval"() -> (w516:dbl)
                    n334 = call-poly <vilib>:"Write Key.vi"("section"=w513, "value"=w516, "key"="Intvl", "refnum"=w515) -> ("refnum out"=w509:T17)  [unwired: 5 in, 2 out]
                    n335 = local read "AVG"() -> (w512:u32)
                    n336 = call-poly <vilib>:"Write Key.vi"("section"=w508, "value"=w512, "key"="Avg", "refnum"=w509) -> ("refnum out"=w510:T17)  [unwired: 5 in, 2 out]
                  }
                  frame True {
                  }
                }
                n337 = local read "Sub1"() -> (w477:enum16{"Off", "Min", "Freq", "Temp", "Res"})
                n338 = local read "Sub2"() -> (w478:enum16{"Off", "Max", "Ratio", "Area", "Second"})
                n339 = local read "Samples"() -> (w502:u32)
                n340 = call-poly <vilib>:"Write Key.vi"("section"=w472, "value"=w502, "key"="Samp", "refnum"=w500) -> ("refnum out"=w487:T17)  [unwired: 5 in, 2 out]
                n341 = local read "LTM"() -> (w471:bool)
                n342 = local read "Int."() -> (w494:i32)
                n343 = call-poly <vilib>:"Write Key.vi"("section"=w472, "value"=w494, "key"="Int", "refnum"=w487) -> ("refnum out"=w488:T17)  [unwired: 5 in, 2 out]
                n344 = call "Write_PanelBounds.vi"("refnum in"=w488, "path"=w489) -> ("refnum out"=w486:T17)
                n345 = call-poly <vilib>:"Write Key.vi"("section"=w483, "value"=w479, "key"="Main", "refnum"=w486) -> ("refnum out"=w485:T17)  [unwired: 5 in, 2 out]
                n346 = call-poly <vilib>:"Write Key.vi"("section"=w483, "value"=w477, "key"="Sub1", "refnum"=w485) -> ("refnum out"=w484:T17)  [unwired: 5 in, 2 out]
                n347 = call-poly <vilib>:"Write Key.vi"("section"=w483, "value"=w478, "key"="Sub2", "refnum"=w484) -> ("refnum out"=w474:T17)  [unwired: 5 in, 2 out]
                n348 = call-poly <vilib>:"Write Key.vi"("section"=w472, "value"=w471, "key"="LTM", "refnum"=w474) -> ("refnum out"=w473:T17)  [unwired: 5 in, 2 out]
                n349 = call <vilib>:"Close Config Data.vi"("refnum"=w473) -> ()  [unwired: 9 in, 2 out]
              }
            }
            n350 = local write "Button8"(w468) -> ()
            n351 = Quit LabVIEW(quit? (T)=w467) -> ()
          }
        }
      }
    }
  }
  n352 = while {
    shift-right: [w518] -> _
    shift-left: StateMachine."Initialize" ("Beginning State") -> [w519]
    stop <- w520 stop-if-true
    n353 = case shown="\"200\"" w519 {
      tunnel: [w529 w653 StateMachine."100" ("Beginning State") w866 w1161 w1482 w1581 w1845 StateMachine."100" ("Beginning State") StateMachine."100" ("Beginning State") w2015 StateMachine."100" ("Beginning State") StateMachine."100" ("Beginning State") StateMachine."100" ("Beginning State") StateMachine."Stop" ("Beginning State")] -> w518
      frame "Initialize", Default {
        w521 = FALSE ("Visible")
        w523 = 1.0 ("X Scale.Range:Minimum")
        w524 = 100.0 ("X Scale.Range:Maximum")
        w525 = dbl[] [] ("History Data")
        w526 = u32 0 ("N2")
        w532 = FALSE ("File?")
        n354 = flat-sequence {
          tunnel: [w598] -> w527
          frame #0 {
            w544 = 1
            w552 = "B" ("section")
            w541 = "A" ("section")
            # "Load Config File"
            n355 = property class="App"() -> ("App.Kind"=w537:T20)  [unwired: 2 in, 2 out]
            n356 = case shown="\"Development System\", Default" w537 {
              tunnel: [w590 w596] -> w536
              tunnel: [w589 w597] -> w535
              frame "Development System", Default {
                n357 = Current VI's Path() -> (path=w589:path)
                n358 = Strip Path(path=w589) -> (stripped path=w590:path)  [unwired: 1 out]
              }
              frame "Run Time System" {
                n359 = Current VI's Path() -> (path=w597:path)
                n360 = Open Application Reference() -> (0:w595:errorcluster, 3:w594:refnum<vi>)  [unwired: 4 in]
                n361 = property class="App"(reference=w594, error in=w595) -> (reference out=w592:refnum<vi>, error out=w593:errorcluster, "App.Dir"=w596:path)
                n362 = Close Reference(reference=w592, error in (no error)=w593) -> (error out=w591:errorcluster)
                n363 = call <vilib>:"Simple Error Handler.vi"("error in (no error)"=w591) -> ()  [unwired: 4 in, 5 out]
              }
            }
            n364 = Build Path(base path=w536, name or relative path="PM100D-ini.cfg") -> (appended path=w571:path)
            n365 = call <vilib>:"Open Config Data (compatibility).vi"("configuration file path"=w571) -> ("error out"=w580:errorcluster, "refnum"=w588:T17)  [unwired: 8 in, 1 out]
            n366 = call-poly <vilib>:"Read Key.vi"("section"=w541, "error in (no error)"=w580, "default value"=4, "key"="Digits", "refnum"=w588) -> ("error out"=w579:errorcluster, "value"=w576:i32, "refnum out"=w585:T17)  [unwired: 3 in, 1 out]
            n367 = local write "Digits"(w576) -> ()
            n368 = call-poly <vilib>:"Read Key.vi"("section"=w541, "error in (no error)"=w579, "default value"=1000.0, "key"="Intvl", "refnum"=w585) -> ("error out"=w578:errorcluster, "value"=w575:dbl, "refnum out"=w583:T17)  [unwired: 3 in, 1 out]
            n369 = local write "Interval"(w575) -> ()
            n370 = call-poly <vilib>:"Read Key.vi"("section"=w541, "error in (no error)"=w578, "default value"=100, "key"="Samp", "refnum"=w583) -> ("error out"=w577:errorcluster, "value"=w574:i32, "refnum out"=w582:T17)  [unwired: 3 in, 1 out]
            n371 = local write "Samples"(w574) -> ()
            n372 = call-poly <vilib>:"Read Key.vi"("section"=w541, "error in (no error)"=w577, "default value"=100, "key"="Avg", "refnum"=w582) -> ("error out"=w568:errorcluster, "value"=w573:i32, "refnum out"=w570:T17)  [unwired: 3 in, 1 out]
            n373 = local write "AVG"(w573) -> ()
            n374 = local read "LTM"() -> (w538:bool)
            n375 = call-poly <vilib>:"Read Key.vi"("section"=w541, "error in (no error)"=w568, "default value"=10, "key"="Int", "refnum"=w570) -> ("error out"=w569:errorcluster, "value"=w566:i32, "refnum out"=w565:T17)  [unwired: 3 in, 1 out]
            n376 = call "Read_PanelBounds.vi"("bot"=720, "top"=100, "right"=1170, "left"=200, "path"=w535, "refnum in"=w565) -> ("refnum out"=w555:T17)  [unwired: 5 in]
            n377 = call-poly <vilib>:"Read Key.vi"("section"=w552, "default value"=0, "key"="Main", "refnum"=w555) -> ("value"=w545:i32, "refnum out"=w554:T17)  [unwired: 4 in, 2 out]
            n378 = local write "MainUnits"(w545) -> ()
            n379 = call-poly <vilib>:"Read Key.vi"("section"=w552, "default value"=w544, "key"="Sub1", "refnum"=w554) -> ("value"=w546:i32, "refnum out"=w553:T17)  [unwired: 4 in, 2 out]
            n380 = local write "Sub1"(w546) -> ()
            n381 = call-poly <vilib>:"Read Key.vi"("section"=w552, "default value"=w544, "key"="Sub2", "refnum"=w553) -> ("value"=w547:i32, "refnum out"=w543:T17)  [unwired: 4 in, 2 out]
            n382 = local write "Sub2"(w547) -> ()
            n383 = call-poly <vilib>:"Read Key.vi"("section"=w541, "default value"=w538, "key"="LTM", "refnum"=w543) -> ("value"=w539:bool, "refnum out"=w542:T17)  [unwired: 4 in, 2 out]
            n384 = local write "LTM"(w539) -> ()
            n385 = local write "Int."(w566) -> ()
            n386 = local write "VI_Path"(w536) -> ()
            n387 = call <vilib>:"Close Config Data.vi"("error in (no error)"=w569, "refnum"=w542) -> ()  [unwired: 8 in, 2 out]
          }
          frame #1 {
            # "Chose Instrument \nand Initialize"
            n388 = call "PM100D_Initialize.vi"() -> ("error out"=w599:errorcluster, "Instrument"=w601:string, "VISA out"=w602:refnum<visa-resource-name>, 4:w600)  [unwired: 2 in]
            n389 = local write "PM100D"(w602) -> ()
            n390 = local write "Flag0"(w601) -> ()
            n391 = local write "Flag1"(w600) -> ()
            n392 = Unbundle By Name(w599) -> ("status"=w598:bool)
          }
        }
        n393 = local write "Button6"(w532) -> ()
        n394 = local write "Button7"(w532) -> ()
        n395 = local write "File?"(w532) -> ()
        n396 = property on="Chart_P" class="WFChart (strict)"("History Data"=w525, "XScale.Maximum"=w524, "XScale.Minimum"=w523) -> ()  [unwired: 2 in, 2 out]
        n397 = local write "Range Array"(string[] ["AUTO", "50nA", "500nA", "5uA", "50uA", "500uA", "5mA"] ("Range Array")) -> ()
        n398 = local write "Frame"(StateMachine."100" ("Frame")) -> ()
        n399 = local write "N2"(w526) -> ()
        n400 = local write "N"(w526) -> ()
        n401 = property on="Chart_E" class="WFChart (strict)"("History Data"=w525, "XScale.Maximum"=w524, "XScale.Minimum"=w523) -> ()  [unwired: 2 in, 2 out]
        n402 = property on="Splitter" class="Splitter"("Position"=285 ("Splitter Position")) -> ()  [unwired: 2 in, 2 out]
        n403 = property on="YT" class="XYGraph (strict)"("Visible"=w521) -> ()  [unwired: 2 in, 2 out]
        n404 = property on="YT" class="XYGraph (strict)"("Value"=cluster{timestamp[], dbl[]} {[timestamp(3408217200 s since 1904-01-01)], []} ("YT")) -> ()  [unwired: 2 in, 2 out]
        n405 = property on="Chart_P" class="WFChart (strict)"("Visible"=w521) -> ()  [unwired: 2 in, 2 out]
        n406 = Select(t=StateMachine."Stop", s=w527, f=StateMachine."Load Settings" ("Beginning State")) -> (s? t:f=w529:T1)
      }
      frame "Load Settings" {
        n407 = local read "PM100D"() -> (w726:refnum<visa-resource-name>)
        n408 = local read "Flag0"() -> (w641:string)
        n409 = local read "LTM"() -> (w648:bool)
        n410 = Spreadsheet String To Array(delimiter (Tab)=",", format string="%s", spreadsheet string=w641, array type (2D Dbl)=string[] [] ("Rng_Array")) -> (array=w642:string[])
        n411 = call "PM100D_Read.vi"("Command"="SYST:SENS:IDN?", "VISA in"=w726) -> ("error out"=w652:errorcluster, "ReadValue"=w669:string, "VISA out"=w691:refnum<visa-resource-name>)  [unwired: 2 in]
        n412 = Index Array(array=w642, index #1=1 ("index"), index #2=2 ("index"), index #3=3 ("index")) -> (element #1=w635:string, element #2=w637:string, element #3=w636:string)
        n413 = Match Pattern(string=w635, regular expression="PM") -> (match substring=w631:string, after substring=w634:string)  [unwired: 1 in, 2 out]
        n414 = Scan String For Tokens(9:w634) -> (1:w632:string)  [unwired: 5 in, 3 out]
        n415 = Concatenate Strings(w631, w632) -> (w629:string)
        n416 = Equal?(x=w629, y="PM100USB") -> (x = y?=w646:bool)
        n417 = Equal?(x=w629, y="PM200") -> (x = y?=w627:bool)
        n418 = Select(t=FALSE, s=w646, f=w648) -> (s? t:f=w650:bool)
        n419 = local write "LTM"(w650) -> ()
        n420 = Not(x=w646) -> (.not. x?=w647:bool)
        n421 = call <vilib>:"Clear Errors.vi"("error in (no error)"=w652) -> ()  [unwired: 5 in, 2 out]
        n422 = Unbundle By Name(w652) -> ("status"=w654:bool)
        n423 = case shown="True" w627 {
          tunnel: [FALSE w730] -> w626
          frame False {
            n424 = local write "EMM"(FALSE ("EMM")) -> ()
          }
          frame True {
            n425 = local read "PM100D"() -> (w734:refnum<visa-resource-name>)
            n426 = call "PM100D_Read.vi"("Command"="SENS3:TEMP:DATA?" ("write buffer"), "VISA in"=w734) -> ("error out"=w729:errorcluster, "ReadValue"=w732:string)  [unwired: 2 in, 1 out]
            n427 = call <vilib>:"Clear Errors.vi"("error in (no error)"=w729) -> ()  [unwired: 5 in, 2 out]
            n428 = Not Equal?(x=w732, y="") -> (x != y?=w730:bool)
            n429 = local write "EMM"(w730) -> ()
          }
        }
        n430 = property on="LTM" class="Bool (strict)"("Visible"=w647) -> ()  [unwired: 2 in, 2 out]
        n431 = Temporary Directory() -> (w615:path)
        n432 = call "PM100D_GetRngIndex.vi"("VISA in"=w691) -> ("error out"=w693:errorcluster, "SensType"=w680:i32, "Rng_Array"=w692:string[], "dup VISA session"=w694:refnum<visa-resource-name>, "IndexOut"=w689:i32, "AutoOut"=w685:bool)  [unwired: 5 in]
        n433 = Build Path(base path=w615, name or relative path="PM_LogData.txt") -> (appended path=w624:path)
        n434 = Equal?(x=3, y=w680) -> (x = y?=w684:bool)
        n435 = Spreadsheet String To Array(delimiter (Tab)=",", format string="%s", spreadsheet string=w669, array type (2D Dbl)=string[] [] ("Rng_Array")) -> (array=w718:string[])
        n436 = case shown="True" w684 {
          tunnel: ["W" ("input 2") "J" ("t")] -> w683
          tunnel: ["POW" ("t") "ENER" ("t")] -> w682
          tunnel: [w802 u32 1 ("AVG")] -> w670
          tunnel: [w801 60000.0 ("x")] -> w665
          frame False {
            n437 = local read "AVG"() -> (w802:u32)
            n438 = local read "Interval"() -> (w801:dbl)
          }
          frame True {
          }
        }
        n439 = Open/Create/Replace File(file path (use dialog)=w624, operation (0:open)=T3."replace or create") -> (refnum out=w620:refnum<file>)  [unwired: 4 in, 2 out]
        n440 = call "PM100D_SetRngIndex.vi"("VISAin"=w694, "Unit"=w682, "AUTO"=w685, "error in"=w693, "SensType"=w680, "Rng_Array"=w692, "Index"=w689) -> ("VISAout"=w690:refnum<visa-resource-name>, "lblRange"=w686:string, "Numeric 2"=w688:dbl, "AUTO?"=w687:bool, "error out 2"=w659:errorcluster)  [unwired: 4 in]
        n441 = Index Array(array=w718, index #1=0 ("index"), index #2=1 ("index"), index #3=4 ("index"), index #4=5 ("index")) -> (element #1=w679:string, element #2=w713:string, element #3=w676:string, element #4=w674:string)
        n442 = Format Into String(format string="%s  SN:%s  Firmware: %s -- Sensor: %s  SN:%s", initial string="", w629, w637, w636, w679, w713) -> (resulting string=w617:string)  [unwired: 1 in, 1 out]
        n443 = local write "Header"(w617) -> ()
        n444 = Concatenate Strings(w617, "\r\n") -> (w618:string)
        n445 = Write to Text File(file (use dialog)=w620, text=w618) -> (refnum out=w619:refnum<file>)  [unwired: 2 in, 2 out]
        n446 = local write "FileRefnum"(w619) -> ()
        n447 = Refnum to Path(1:w619) -> (0:w622:path)
        n448 = Equal?(x=w679, y="no sensor") -> (x = y?=w655:bool)
        n449 = call "PM100D_SensIDNFlag.vi"("String"=w674) -> ("Wave?"=w616:bool, "Tau?"=w671:bool, "Temp?"=w673:bool)  [unwired: 4 out]
        n450 = local write "Wav"(w616) -> ()
        n451 = local write "LFP"(w622) -> ()
        n452 = Format Into String(format string="%s%s", initial string="Range ", w686, w683) -> (resulting string=w711:string)  [unwired: 1 in, 1 out]
        n453 = Divide(x=1000.0, y=w688) -> (x/y=w706:dbl)
        n454 = Or(x=w655, y=w654) -> (x .or. y?=w656:bool)
        n455 = Not Equal?(x=w676, y="1") -> (x != y?=w672:bool)
        n456 = local write "SlideMulti"(w706) -> ()
        n457 = property on="Button1" class="Bool (strict)"("BoolText.Text"=w711) -> ()  [unwired: 2 in, 2 out]
        n458 = case shown="True" w656 {
          tunnel: [StateMachine."20" ("Beginning State") w737] -> w653
          frame False {
          }
          frame True {
            n459 = call "Dialog_NoSensor.vi"() -> ("Cancel"=w739:bool)  [unwired: 5 in, 1 out]
            n460 = Select(t=StateMachine."Load Settings", s=w739, f=StateMachine."Stop" ("Beginning State")) -> (s? t:f=w737:T1)
          }
        }
        n461 = local write "Temp"(w673) -> ()
        n462 = local write "Sensor?"(w672) -> ()
        n463 = local write "Tau?"(w671) -> ()
        n464 = local write "AUTO?"(w687) -> ()
        n465 = local write "SensType"(w680) -> ()
        n466 = property on="EMM" class="Bool (strict)"("Visible"=w626) -> ()  [unwired: 2 in, 2 out]
        n467 = local read "Samples"() -> (w702:u32)
        n468 = local read "File?"() -> (w701:bool)
        n469 = Format Into String(format string="%d", initial string="SENS:AVER " ("Command"), w670) -> (resulting string=w695:string)  [unwired: 1 in, 1 out]
        n470 = property on="Hum" class="Str"("Visible"=w626) -> ()  [unwired: 2 in, 2 out]
        n471 = local write "AVG"(w670) -> ()
        n472 = call "PM100D_Write.vi"("error in (no error)"=w659, "Command"=w695, "VISA in"=w690) -> ("error out"=w658:errorcluster, "VISA out"=w698:refnum<visa-resource-name>)
        n473 = call "PM100D_Read.vi"("error in (no error)"=w658, "Command"="SENS:CORR:BEAM?", "VISA in"=w698) -> ("error out"=w657:errorcluster, "ReadValue"=w721:string, "VISA out"=w720:refnum<visa-resource-name>)  [unwired: 1 in]
        n474 = case shown="1" w680 {
          tunnel: w720 -> [w741 w748 w780 w792]
          tunnel: [w741 w746 w771 w791] -> w614
          tunnel: w657 -> [w740 w745 w770 w790]
          tunnel: [w740 w744 w769 w789] -> w611
          frame 0, Default {
          }
          frame 1 {
            n475 = local read "MainUnits"() -> (w743:enum16{"W", "V", "J", "dBm", "A"})
            n476 = call "PM100D_Read.vi"("error in (no error)"=w745, "Command"="INP:FILT?", "VISA in"=w748) -> ("error out"=w744:errorcluster, "ReadValue"=w749:string, "VISA out"=w746:refnum<visa-resource-name>)  [unwired: 1 in]
            n477 = case shown="\"A\"" w743 {
              tunnel: [enum16{"W", "V", "J", "dBm", "A"}."W" ("MainUnits") enum16{"W", "V", "J", "dBm", "A"}."W" ("MainUnits") enum16{"W", "V", "J", "dBm", "A"}."W" ("MainUnits") enum16{"W", "V", "J", "dBm", "A"}."dBm" ("MainUnits") enum16{"W", "V", "J", "dBm", "A"}."A" ("MainUnits")] -> w742
              frame "W", Default {
              }
              frame "V" {
              }
              frame "J" {
              }
              frame "dBm" {
              }
              frame "A" {
              }
            }
            n478 = Decimal String To Number(string=w749) -> (number=w747:i32)  [unwired: 2 in, 1 out]
            n479 = local write "MainUnits"(w742) -> ()
            n480 = local write "BW"(w747) -> ()
          }
          frame 2 {
            w762 = "1\n" ("y")
            n481 = call "PM100D_Read.vi"("error in (no error)"=w770, "Command"="INP:THER:ACC?", "VISA in"=w780) -> ("error out"=w767:errorcluster, "ReadValue"=w779:string, "VISA out"=w768:refnum<visa-resource-name>)  [unwired: 1 in]
            n482 = call "PM100D_Read.vi"("error in (no error)"=w767, "Command"="INP:THER:ACC:AUTO?", "VISA in"=w768) -> ("error out"=w764:errorcluster, "ReadValue"=w763:string, "VISA out"=w765:refnum<visa-resource-name>)  [unwired: 1 in]
            n483 = call "PM100D_Read.vi"("error in (no error)"=w764, "Command"="INP:THER:ACC:TAU?", "VISA in"=w765) -> ("error out"=w769:errorcluster, "ReadValue"=w773:string, "VISA out"=w771:refnum<visa-resource-name>)  [unwired: 1 in]
            n484 = Equal?(x=w779, y=w762) -> (x = y?=w778:bool)
            n485 = Equal?(x=w763, y=w762) -> (x = y?=w761:bool)
            n486 = Select(t="ON", s=w778, f="OFF") -> (s? t:f=w758:string)
            n487 = Fract/Exp String To Number(use system decimal point (T)=FALSE, string=w773) -> (number=w772:dbl)  [unwired: 2 in, 1 out]
            n488 = local read "MainUnits"() -> (w756:enum16{"W", "V", "J", "dBm", "A"})
            n489 = local write "Tau"(w772) -> ()
            n490 = Select(t="AUTO", s=w761, f=w758) -> (s? t:f=w759:string)
            n491 = local write "ACC"(w759) -> ()
            n492 = case shown="\"J\"" w756 {
              tunnel: [enum16{"W", "V", "J", "dBm", "A"}."W" ("MainUnits") enum16{"W", "V", "J", "dBm", "A"}."V" ("MainUnits") enum16{"W", "V", "J", "dBm", "A"}."W" ("MainUnits") enum16{"W", "V", "J", "dBm", "A"}."dBm" ("MainUnits") enum16{"W", "V", "J", "dBm", "A"}."W" ("MainUnits")] -> w757
              frame "W", Default {
              }
              frame "V" {
              }
              frame "J" {
              }
              frame "dBm" {
              }
              frame "A" {
              }
            }
            n493 = local write "MainUnits"(w757) -> ()
          }
          frame 3 {
            n494 = local read "MainUnits"() -> (w788:enum16{"W", "V", "J", "dBm", "A"})
            n495 = call "PM100D_Read.vi"("error in (no error)"=w790, "Command"="SENS:PEAK?", "VISA in"=w792) -> ("error out"=w789:errorcluster, "ReadValue"=w794:string, "VISA out"=w791:refnum<visa-resource-name>)  [unwired: 1 in]
            n496 = case shown="\"W\", Default" w788 {
              tunnel: [enum16{"W", "V", "J", "dBm", "A"}."J" ("MainUnits") enum16{"W", "V", "J", "dBm", "A"}."V" ("MainUnits") enum16{"W", "V", "J", "dBm", "A"}."J" ("MainUnits") enum16{"W", "V", "J", "dBm", "A"}."J" ("MainUnits") enum16{"W", "V", "J", "dBm", "A"}."J" ("MainUnits")] -> w787
              frame "W", Default {
              }
              frame "V" {
              }
              frame "J" {
              }
              frame "dBm" {
              }
              frame "A" {
              }
            }
            n497 = Fract/Exp String To Number(string=w794) -> (number=w795:dbl)  [unwired: 3 in, 1 out]
            n498 = local write "Trig"(w795) -> ()
            n499 = local write "MainUnits"(w787) -> ()
          }
        }
        n500 = property on="Temp" class="Str"("Visible"=w626) -> ()  [unwired: 2 in, 2 out]
        n501 = Divide(x=w665, y=1000.0) -> (x/y=w699:dbl)
        n502 = Fract/Exp String To Number(use system decimal point (T)=FALSE, string=w721) -> (number=w630:dbl)  [unwired: 2 in, 1 out]
        n503 = call "PM100D_Read.vi"("error in (no error)"=w611, "Command"="SENS:CORR?", "VISA in"=w614) -> ("error out"=w612:errorcluster, "ReadValue"=w607:string, "VISA out"=w613:refnum<visa-resource-name>)  [unwired: 1 in]
        n504 = call "PM100D_Read.vi"("error in (no error)"=w612, "Command"="INP:ADAP?", "VISA in"=w613) -> ("error out"=w660:errorcluster, "ReadValue"=w663:string)  [unwired: 1 in, 1 out]
        n505 = Format Into String(format string="Samples:    %d\\nInterval:      %.2fs\\nAveraging: %d\\nLog to File: %s", initial string="Logging Parameters\n", w702, w699, w670, w701) -> (resulting string=w703:string)  [unwired: 1 in, 1 out]
        n506 = local write "Dia"(w630) -> ()
        n507 = local write "LogCfg"(w703) -> ()
        n508 = Search 1D Array(1D array=string[] ["PHOT\n", "THER\n", "PYR\n"], element=w663) -> (index of element=w662:i32)  [unwired: 1 in]
        n509 = local write "DiaIni"(w630) -> ()
        n510 = local write "Adapter"(w662) -> ()
        n511 = Fract/Exp String To Number(use system decimal point (T)=FALSE, string=w607) -> (number=w603:dbl)  [unwired: 2 in, 1 out]
        n512 = local write "Readout"("   ---   " ("Readout")) -> ()
        n513 = local write "Sub1"("Min:     ---   " ("Sub1")) -> ()
        n514 = local write "Sub2"("Max:     ---   " ("Sub2")) -> ()
        n515 = local write "Att"(w603) -> ()
        n516 = Format Into String(format string="%.;%.2f %s", initial string="a = ", w603, " dB") -> (resulting string=w605:string)  [unwired: 1 in, 1 out]
        n517 = call <vilib>:"Clear Errors.vi"("error in (no error)"=w660) -> ()  [unwired: 5 in, 2 out]
        n518 = local write "att"(w605) -> ()
      }
      frame "20" {
        n519 = local read "PM100D"() -> (w814:refnum<visa-resource-name>)
        n520 = local read "SensType"() -> (w809:i32)
        n521 = local read "Sensor?"() -> (w813:bool)
        n522 = local read "MainUnits"() -> (w811:enum16{"W", "V", "J", "dBm", "A"})
        n523 = case shown="True" w813 {
          tunnel: [w836 "Wave " ("initial string")] -> w821
          tunnel: [w835 "%dnm" ("format string")] -> w820
          tunnel: [w839 w859] -> w819
          tunnel: [1e-07 ("WAV_MAX") w858] -> w818
          tunnel: [1000.0 ("WAV_MAX") w857] -> w817
          tunnel: w814 -> [w834 w856]
          tunnel: w809 -> [w833 _]
          tunnel: [w832 w855] -> w812
          frame False {
            # "CORR:POW?\nCORR:POW:THER?\nCORR:ENER?"
            n524 = case shown="0, Default" w833 {
              tunnel: ["" ("format string") "SENS:CORR:POW?" ("format string") "SENS:CORR:POW:THER?" ("format string") "SENS:CORR:ENER?" ("format string")] -> w837
              tunnel: ["" ("initial string") "" ("initial string") "" ("initial string") "" ("initial string")] -> w836
              tunnel: ["" ("format string") "%.;%_3pA/W" ("format string") "%.;%_3pV/W" ("format string") "%.;%_3pV/J" ("format string")] -> w835
              frame 0, Default {
              }
              frame 1 {
              }
              frame 2 {
              }
              frame 3 {
              }
            }
            n525 = call "PM100D_Read.vi"("Command"=w837, "VISA in"=w834) -> ("error out"=w832:errorcluster, "ReadValue"=w840:string)  [unwired: 2 in, 1 out]
            n526 = Fract/Exp String To Number(use system decimal point (T)=FALSE, string=w840) -> (number=w839:dbl)  [unwired: 2 in, 1 out]
          }
          frame True {
            n527 = call "PM100D_Get-Wave.vi"("VISA in"=w856) -> ("WAV_MAX"=w857:dbl, "WAV"=w859:dbl, "WAV_MIN"=w858:dbl, "error out"=w855:errorcluster)  [unwired: 10 in, 1 out]
          }
        }
        n528 = case shown="\"V\"" w811 {
          tunnel: ["Power / W" w823 "Energy / J" "dBm" "Power / A"] -> w810
          tunnel: w809 -> [_ w824 _ _ _]
          frame "W", Default {
          }
          frame "V" {
            n529 = case shown="0, Default" w824 {
              tunnel: ["" "Power / V" "Power / V" "Energy / V"] -> w823
              frame 0, Default {
              }
              frame 1 {
              }
              frame 2 {
              }
              frame 3 {
              }
            }
          }
          frame "J" {
          }
          frame "dBm" {
          }
          frame "A" {
          }
        }
        n530 = local write "Unit"(w810) -> ()
        n531 = Format Into String(format string=w820, initial string=w821, w819) -> (resulting string=w816:string)  [unwired: 1 in, 1 out]
        n532 = call <vilib>:"Clear Errors.vi"("error in (no error)"=w812) -> ()  [unwired: 5 in, 2 out]
        n533 = local write "LambdaMax"(w817) -> ()
        n534 = property on="Button2" class="Bool (strict)"("BoolText.Text"=w816) -> ()  [unwired: 2 in, 2 out]
        n535 = local write "LambdaMin"(w818) -> ()
        n536 = local write "Lambda"(w819) -> ()
      }
      frame "100" {
        n537 = flat-sequence {
          tunnel: [w959] -> w865
          tunnel: [w958] -> w864
          tunnel: [w940] -> w863
          tunnel: [w946] -> w862
          frame #0 {
            n538 = local read "MainUnits"() -> (w957:enum16{"W", "V", "J", "dBm", "A"})
            n539 = local read "LTM"() -> (w942:bool)
            n540 = case shown="False" w942 {
              tunnel: [w964 w975] -> w943
              frame False {
                n541 = local read "Wav"() -> (w963:bool)
                n542 = case shown="True" w963 {
                  tunnel: [w970 w972] -> w964
                  frame False {
                    n543 = local read "PM100D"() -> (w971:refnum<visa-resource-name>)
                    n544 = call "PM100D_Get-Wave.vi"("VISA in"=w971) -> ("VISA out"=w970:refnum<visa-resource-name>, "WAV"=w967:dbl, "error out"=w965:errorcluster)  [unwired: 10 in, 2 out]
                    n545 = Format Into String(format string="%dnm", initial string="Wave ", w967) -> (resulting string=w966:string)  [unwired: 1 in, 1 out]
                    n546 = local write "Lambda"(w967) -> ()
                    n547 = property on="Button2" class="Bool (strict)"("BoolText.Text"=w966) -> ()  [unwired: 2 in, 2 out]
                    n548 = call <vilib>:"Clear Errors.vi"("error in (no error)"=w965) -> ()  [unwired: 5 in, 2 out]
                  }
                  frame True {
                    n549 = local read "PM100D"() -> (w972:refnum<visa-resource-name>)
                  }
                }
              }
              frame True {
                n550 = local read "PM100D"() -> (w973:refnum<visa-resource-name>)
                n551 = call "PM100D_Open.vi"("VISA resource name"=w973) -> ("VISA out"=w975:refnum<visa-resource-name>, "error out"=w974:errorcluster)  [unwired: 2 out]
                n552 = call <vilib>:"Clear Errors.vi"("error in (no error)"=w974) -> ()  [unwired: 5 in, 2 out]
              }
            }
            n553 = call "PM100D_Read.vi"("Command"="SYST:SENS:IDN?", "VISA in"=w943) -> ("error out"=w944:errorcluster, "ReadValue"=w953:string)  [unwired: 2 in, 1 out]
            n554 = case shown="\"V\"" w957 {
              tunnel: ["VOLT" ("ConfPara") "ENER" ("ConfPara") "POW" ("ConfPara") "CURR" ("ConfPara") "POW" ("ConfPara")] -> w958
              tunnel: ["V" "J" "dBm" "A" "W"] -> w941
              frame "V" {
              }
              frame "J" {
              }
              frame "dBm" {
              }
              frame "A" {
              }
              frame "W", Default {
              }
            }
            n555 = local write "Button7"(FALSE ("Button7")) -> ()
            n556 = local read "SensType"() -> (w956:i32)
            n557 = Unbundle By Name(w944) -> ("status"=w947:bool)
            n558 = xnode "Match Regular Expression"("input string"=w953, "regular expression"=",") -> ("before match"=w950:string)  [unwired: 4 in, 4 out]
            n559 = local read "PM100D"() -> (w959:refnum<visa-resource-name>)
            n560 = Equal?(x="no sensor" ("y"), y=w950) -> (x = y?=w948:bool)
            n561 = Or(x=w947, y=w948) -> (x .or. y?=w949:bool)
            n562 = case shown="True" w949 {
              tunnel: [FALSE w977] -> w946
              frame False {
              }
              frame True {
                n563 = disable-structure shown="Enabled" {
                  disable-tunnel: [w978 TRUE ("OK")] -> w977
                  frame Disabled {
                    n564 = call "Dialog_LostConnection.vi"() -> ("OK"=w978:bool)  [unwired: 7 in]
                  }
                  frame Enabled {
                  }
                }
              }
            }
            n565 = call <vilib>:"Clear Errors.vi"("error in (no error)"=w944) -> ()  [unwired: 5 in, 2 out]
            n566 = Equal?(x=w956, y=3) -> (x = y?=w940:bool)
            n567 = case shown="True" w940 {
              tunnel: [0 2] -> w939
              frame False {
              }
              frame True {
                n568 = property on="YT" class="XYGraph (strict)"("Visible"=FALSE) -> ()  [unwired: 2 in, 2 out]
              }
            }
            n569 = property on="Scale" class="Bool (strict)"("Disabled"=w939) -> ()  [unwired: 2 in, 2 out]
            n570 = local write "Unt"(w941) -> ()
          }
        }
        n571 = case shown="False" w862 {
          tunnel: [w870 StateMachine."Load Settings" ("Frame")] -> w866
          tunnel: w865 -> [w868 w937]
          tunnel: w864 -> [w869 _]
          tunnel: w863 -> [w867 _]
          frame False {
            n572 = case shown="True" w867 {
              tunnel: [w872 w903] -> w870
              tunnel: w869 -> [w886 w902]
              tunnel: w867 -> [_ w897]
              tunnel: w868 -> [w887 w895]
              frame False {
                w875 = 0 ("t")
                w874 = 2
                n573 = local read "FastOut"() -> (w883:bool)
                n574 = local read "Button6"() -> (w882:bool)
                n575 = Concatenate Strings("CONF:" ("string"), w886) -> (w889:string)
                n576 = And(x=w883, y=w882) -> (x .and. y?=w881:bool)
                n577 = local read "XScaleFit"() -> (w873:bool)
                n578 = local read "YScaleFit"() -> (w878:bool)
                n579 = local read "YScaleRep"() -> (w877:bool)
                n580 = call "PM100D_Write.vi"("Command"=w889, "VISA in"=w887) -> ("error out"=w871:errorcluster)  [unwired: 1 in, 1 out]
                n581 = case shown="True" w881 {
                  tunnel: [StateMachine."120" ("Frame") StateMachine."130" ("Frame")] -> w872
                  frame False {
                  }
                  frame True {
                    w892 = "---" ("Sub1")
                    n582 = local write "Sub1"(w892) -> ()
                    n583 = local write "Sub2"(w892) -> ()
                    n584 = local write "Readout"("- Acquiring -" ("Readout")) -> ()
                    n585 = local write "Stat0"("Count:" ("Stat0")) -> ()
                  }
                }
                n586 = call <vilib>:"Clear Errors.vi"("error in (no error)"=w871) -> ()  [unwired: 5 in, 2 out]
                n587 = Select(t=w875, s=w873, f=w874) -> (s? t:f=w876:i32)
                n588 = Select(t=w875, s=w878, f=w874) -> (s? t:f=w880:i32)
                n589 = Boolean To (0,1)(Boolean=w877) -> (0, 1=w879:i16)
                n590 = property on="Chart_P" class="WFChart (strict)"("XScale.ScaleFit"=w876, "YScale.ScaleFit"=w880, "YScale.Mapping Mode"=w879) -> ()  [unwired: 2 in, 2 out]
                n591 = local write "ARM"(TRUE ("ARM")) -> ()
                n592 = local write "Arm"("T" ("Arm")) -> ()
              }
              frame True {
                n593 = call "PM100D_ConfMeas.vi"("Conf:"=w902, "VISA In"=w895) -> ("error out"=w896:errorcluster, "dup VISA session"=w901:refnum<visa-resource-name>)  [unwired: 1 in]
                n594 = call <vilib>:"Clear Errors.vi"("error in (no error)"=w896) -> ()  [unwired: 5 in, 2 out]
                n595 = while {
                  tunnel: w901 -> [w934]
                  tunnel: [w911] -> w905
                  tunnel: w897 -> [w920]
                  i -> [w923]
                  stop <- w933 stop-if-true
                  n596 = local read "Button1"() -> (w932:bool)
                  n597 = local read "Button2"() -> (w931:bool)
                  n598 = local read "Button3"() -> (w930:bool)
                  n599 = local read "Button4"() -> (w929:bool)
                  n600 = local read "Button5"() -> (w928:bool)
                  n601 = local read "Button8"() -> (w927:bool)
                  n602 = Select(t=10000, s=w920, f=2) -> (s? t:f=w919:i32)
                  n603 = local read "AVG"() -> (w921:u32)
                  n604 = call "PM100D_Read.vi"("Command"="STAT:OPER:COND?", "VISA in"=w934) -> ("error out"=w906:errorcluster, "ReadValue"=w935:string)  [unwired: 2 in, 1 out]
                  n605 = Unbundle By Name(w906) -> ("status"=w907:bool)
                  n606 = Decimal String To Number(string=w935) -> (number=w913:i32)  [unwired: 2 in, 1 out]
                  n607 = Multiply(x=w919, y=w921) -> (x*y=w922:u32)
                  n608 = Number To Boolean Array(number=w913) -> (Boolean array=w910:bool[])
                  n609 = local read "Button9"() -> (w915:bool)
                  n610 = local read "Button10"() -> (w914:bool)
                  n611 = call <vilib>:"Clear Errors.vi"("error in (no error)"=w906) -> ()  [unwired: 5 in, 2 out]
                  n612 = Equal?(x=w923, y=w922) -> (x = y?=w916:bool)
                  n613 = Rotate 1D Array(1:w910, 2:0 ("n")) -> (0:w909:bool[])
                  n614 = Index Array(array=w909, index=9) -> (element=w911:bool)
                  n615 = Select(t="T", s=w911, f="A") -> (s? t:f=w926:string)
                  n616 = Compound Arithmetic op=OR(w907, w911, w932, w931, w930, w929, w928, w927, w916, w915, w914) -> (w933:bool)
                  n617 = local write "ARM"(w911) -> ()
                  n618 = local write "Arm"(w926) -> ()
                }
                n619 = local read "Frame"() -> (w904:T1)
                n620 = Select(t=StateMachine."140", s=w897, f=StateMachine."120" ("t")) -> (s? t:f=w899:T1)
                n621 = Select(t=w899, s=w905, f=w904) -> (s? t:f=w903:T1)
              }
            }
          }
          frame True {
            n622 = call "PM100D_Close.vi"("VISA resource name"=w937) -> ()  [unwired: 3 in]
          }
        }
      }
      frame "120" {
        n623 = local read "PM100D"() -> (w1105:refnum<visa-resource-name>)
        n624 = local read "Digits"() -> (w1146:i32)
        n625 = local read "MainUnits"() -> (w1104:enum16{"W", "V", "J", "dBm", "A"})
        n626 = case shown="\"W\", Default" w1104 {
          tunnel: ["POW?" "ENER?" "VOLT?" "POW?" "CURR?"] -> w1101
          frame "W", Default {
          }
          frame "J" {
          }
          frame "V" {
          }
          frame "dBm" {
          }
          frame "A" {
          }
        }
        n627 = local read "Button6"() -> (w1108:bool)
        n628 = local read "Button7"() -> (w1128:bool)
        n629 = local read "SensType"() -> (w1133:i32)
        n630 = local read "Scale"() -> (w1109:bool)
        n631 = local read "Sub1"() -> (w1153:enum16{"Off", "Min", "Freq", "Temp", "Res"})
        n632 = local read "AVG"() -> (w1134:u32)
        n633 = local read "Sub2"() -> (w1152:enum16{"Off", "Max", "Ratio", "Area", "Second"})
        n634 = local read "N2"() -> (w1111:u32)
        n635 = local read "EMM"() -> (w1112:bool)
        n636 = Increment(x=w1111) -> (x+1=w1110:u32)
        n637 = Concatenate Strings("MEAS:" ("Command"), w1101) -> (w1102:string)
        n638 = Equal?(x=w1133, y=3) -> (x = y?=w1137:bool)
        n639 = local write "N2"(w1110) -> ()
        n640 = case shown="True" w1108 {
          tunnel: w1109 -> [w1170 _]
          frame False {
            n641 = property on="Chart_P" class="WFChart (strict)"("Visible"=w1170) -> ()  [unwired: 2 in, 2 out]
            n642 = Not(x=w1170) -> (.not. x?=w1171:bool)
            n643 = property on="YT" class="XYGraph (strict)"("Visible"=w1171) -> ()  [unwired: 2 in, 2 out]
          }
          frame True {
            n644 = property on="Chart_P" class="WFChart (strict)"("Visible"=TRUE) -> ()  [unwired: 2 in, 2 out]
          }
        }
        n645 = call "PM100D_Read.vi"("Command"=w1102, "VISA in"=w1105) -> ("error out"=w1106:errorcluster, "ReadValue"=w1124:string, "VISA out"=w1116:refnum<visa-resource-name>)  [unwired: 2 in]
        n646 = case shown="True" w1112 {
          frame True {
            n647 = local read "AVG"() -> (w1176:u32)
            n648 = Greater Or Equal?(x=w1176, y=u32 100) -> (x >= y?=w1177:bool)
            n649 = Divide(x=w1176, y=u32 1000) -> (x/y=w1175:dbl)
            n650 = local read "N2"() -> (w1183:u32)
            n651 = Select(t=w1175, s=w1177, f=0.1) -> (s? t:f=w1173:dbl)
            n652 = Divide(x=u32 3 ("y"), y=w1173) -> (x/y=w1179:dbl)
            n653 = Round Toward +Infinity(x=w1179) -> (ceil(x): smallest int >= x=w1180:dbl)
            n654 = Equal?(x=w1183, y=w1180) -> (x = y?=w1184:bool)
            n655 = case shown="False" w1184 {
              frame False {
              }
              frame True {
                n656 = local read "PM100D"() -> (w1196:refnum<visa-resource-name>)
                n657 = call "PM100D_Read.vi"("Command"="SENS3:TEMP:DATA?" ("write buffer"), "VISA in"=w1196) -> ("error out"=w1186:errorcluster, "ReadValue"=w1192:string, "VISA out"=w1195:refnum<visa-resource-name>)  [unwired: 2 in]
                n658 = Equal?(x="", y=w1192) -> (x = y?=w1193:bool)
                n659 = case shown="False" w1193 {
                  tunnel: w1192 -> [w1207 _]
                  frame False {
                    n660 = Fract/Exp String To Number(use system decimal point (T)=FALSE, string=w1207) -> (number=w1203:dbl)  [unwired: 2 in, 1 out]
                    n661 = local write "T"(w1203) -> ()
                    n662 = Format Into String(format string="%.;%.1f\\B0C", w1203) -> (resulting string=w1205:string)  [unwired: 2 in, 1 out]
                    n663 = local write "Temp"(w1205) -> ()
                  }
                  frame True {
                  }
                }
                n664 = call "PM100D_Read.vi"("error in (no error)"=w1186, "Command"="SENS2:HUM:DATA?" ("write buffer"), "VISA in"=w1195) -> ("error out"=w1191:errorcluster, "ReadValue"=w1188:string)  [unwired: 1 in, 1 out]
                n665 = call <vilib>:"Clear Errors.vi"("error in (no error)"=w1191) -> ()  [unwired: 5 in, 2 out]
                n666 = Equal?(x=w1188, y="") -> (x = y?=w1189:bool)
                n667 = case shown="False" w1189 {
                  tunnel: w1188 -> [w1199 _]
                  frame False {
                    n668 = Fract/Exp String To Number(use system decimal point (T)=FALSE, string=w1199) -> (number=w1198:dbl)  [unwired: 2 in, 1 out]
                    n669 = Format Into String(format string="%.;%.1f%", w1198) -> (resulting string=w1201:string)  [unwired: 2 in, 1 out]
                    n670 = local write "Hum"(w1201) -> ()
                    n671 = local write "H"(w1198) -> ()
                  }
                  frame True {
                  }
                }
                n672 = local write "N2"(u32 0 ("N2")) -> ()
              }
            }
          }
          frame False {
          }
        }
        n673 = Unbundle By Name(w1106) -> ("status"=w1107:bool)
        n674 = call <vilib>:"Clear Errors.vi"("error in (no error)"=w1106) -> ()  [unwired: 5 in, 2 out]
        n675 = Equal?(x="9.9E37\n", y=w1124) -> (x = y?=w1122:bool)
        n676 = Equal?(x="-9.9E37\n", y=w1124) -> (x = y?=w1123:bool)
        n677 = Build Array(w1122, w1123) -> (w1121:bool[])
        n678 = Boolean Array To Number(Boolean array=w1121) -> (number=w1120:u32)
        n679 = case shown="0, Default" w1120 {
          tunnel: [w1217 w1255 w1264] -> w1148
          tunnel: w1146 -> [w1216 _ _]
          tunnel: [w1210 w1254 w1263] -> w1139
          tunnel: w1104 -> [w1215 w1256 w1265]
          tunnel: [w1210 w1254 w1263] -> w1132
          tunnel: [w1214 "High     " "Low      "] -> w1127
          tunnel: w1124 -> [w1211 _ _]
          tunnel: [w1209 w1254 w1263] -> w1117
          frame 0, Default {
            n680 = Number To Decimal String(number=w1216) -> (decimal integer string=w1212:string)  [unwired: 1 in]
            n681 = case shown="\"W\", Default" w1215 {
              tunnel: [w1222 w1229 w1236 w1244 w1251] -> w1213
              tunnel: [w1219 w1226 w1233 w1243 w1248] -> w1210
              tunnel: w1212 -> [w1223 w1230 w1237 w1245 w1252]
              tunnel: [w1221 w1228 w1235 w1242 w1250] -> w1217
              tunnel: [w1219 w1226 w1233 w1240 w1248] -> w1209
              tunnel: w1211 -> [w1218 w1225 w1232 w1239 w1247]
              frame "W", Default {
                w1221 = "pW" ("string")
                n682 = Fract/Exp String To Number(use system decimal point (T)=FALSE, string=w1218) -> (number=w1219:dbl)  [unwired: 2 in, 1 out]
                n683 = Concatenate Strings("%.;%_" ("string"), w1223, w1221) -> (w1222:string)
              }
              frame "V" {
                w1228 = "pV" ("string")
                n684 = Fract/Exp String To Number(use system decimal point (T)=FALSE, string=w1225) -> (number=w1226:dbl)  [unwired: 2 in, 1 out]
                n685 = Concatenate Strings("%.;%_" ("string"), w1230, w1228) -> (w1229:string)
              }
              frame "J" {
                w1235 = "pJ" ("string")
                n686 = Fract/Exp String To Number(use system decimal point (T)=FALSE, string=w1232) -> (number=w1233:dbl)  [unwired: 2 in, 1 out]
                n687 = Concatenate Strings("%.;%_" ("string"), w1237, w1235) -> (w1236:string)
              }
              frame "dBm" {
                w1242 = "fdBm" ("string")
                n688 = Fract/Exp String To Number(use system decimal point (T)=FALSE, string=w1239) -> (number=w1240:dbl)  [unwired: 2 in, 1 out]
                n689 = call "lin-log.vi"("W In 2"=w1240) -> ("dBm Out 2"=w1243:dbl)  [unwired: 3 in, 3 out]
                n690 = Concatenate Strings("%.;%_" ("string"), w1245, w1242) -> (w1244:string)
              }
              frame "A" {
                w1250 = "pA" ("string")
                n691 = Fract/Exp String To Number(use system decimal point (T)=FALSE, string=w1247) -> (number=w1248:dbl)  [unwired: 2 in, 1 out]
                n692 = Concatenate Strings("%.;%_" ("string"), w1252, w1250) -> (w1251:string)
              }
            }
            n693 = Format Into String(format string=w1213, w1210) -> (resulting string=w1214:string, error out=w1208:errorcluster)  [unwired: 2 in]
            n694 = call <vilib>:"Clear Errors.vi"("error in (no error)"=w1208) -> ()  [unwired: 5 in, 2 out]
          }
          frame 1 {
            w1254 = 0.0
            n695 = case shown="\"dBm\"" w1256 {
              tunnel: ["W" ("string") "V" ("string") "J" ("string") "A" ("string") "dBm" ("string")] -> w1255
              frame "W", Default {
              }
              frame "V" {
              }
              frame "J" {
              }
              frame "A" {
              }
              frame "dBm" {
              }
            }
          }
          frame 2 {
            w1263 = 0.0
            n696 = case shown="\"A\"" w1265 {
              tunnel: ["W" ("string") "V" ("string") "J" ("string") "A" ("string") "dBm" ("string")] -> w1264
              frame "W", Default {
              }
              frame "V" {
              }
              frame "J" {
              }
              frame "A" {
              }
              frame "dBm" {
              }
            }
          }
        }
        n697 = call <vilib>:"Array Max & Min PtByPt.vi"("input data point"=w1132, "sample length"=0, "initialize"=w1128) -> ("max value"=w1150:dbl, "min value"=w1149:dbl)  [unwired: 3 out]
        n698 = case shown="\"Freq\"" w1153 {
          tunnel: ["%d" "%.;%_6fHz" "%.;%_3f°C" "%.;%d Ohm" w1458] -> w1160
          tunnel: ["" "f: " "T: " "R: " "Min:  "] -> w1158
          tunnel: [0.0 ("min value") w1411 w1431 w1451 w1462] -> w1155
          tunnel: w1149 -> [_ _ _ _ w1462]
          tunnel: w1148 -> [w1393 w1414 w1434 w1454 w1459]
          tunnel: [w1393 w1414 w1434 w1454 w1459] -> w1147
          tunnel: w1116 -> [w1392 w1409 w1429 w1449 w1457]
          tunnel: w1134 -> [_ w1403 w1423 w1443 _]
          tunnel: [w1392 w1401 w1421 w1441 w1457] -> w1115
          frame "Off", Default {
            (unwired) FALSE
          }
          frame "Freq" {
            (unwired) FALSE
            n699 = call "PM100D_Write.vi"("Command"="SENS:AVER 1", "VISA in"=w1409) -> ("error out"=w1400:errorcluster, "VISA out"=w1408:refnum<visa-resource-name>)  [unwired: 1 in]
            n700 = call "PM100D_Meas.vi"("error in"=w1400, "Timeout"=500 ("Aver"), "ConfPara"="FREQ", "VISA Out"=w1408) -> ("error out"=w1399:errorcluster, "ReadValue"=w1413:string, "dup VISA session"=w1406:refnum<visa-resource-name>)  [unwired: 1 out]
            n701 = Format Into String(format string="SENS:AVER %d", error in=w1399, w1403) -> (resulting string=w1404:string, error out=w1398:errorcluster)  [unwired: 1 in]
            n702 = call "PM100D_Write.vi"("error in (no error)"=w1398, "Command"=w1404, "VISA in"=w1406) -> ("error out"=w1397:errorcluster, "VISA out"=w1401:refnum<visa-resource-name>)
            n703 = Fract/Exp String To Number(use system decimal point (T)=FALSE, string=w1413) -> (number=w1411:dbl)  [unwired: 2 in, 1 out]
            n704 = call <vilib>:"Clear Errors.vi"("error in (no error)"=w1397) -> ()  [unwired: 5 in, 2 out]
          }
          frame "Temp" {
            n705 = call "PM100D_Write.vi"("Command"="SENS:AVER 1", "VISA in"=w1429) -> ("error out"=w1420:errorcluster, "VISA out"=w1428:refnum<visa-resource-name>)  [unwired: 1 in]
            n706 = call "PM100D_Meas.vi"("error in"=w1420, "Timeout"=10 ("Aver"), "ConfPara"="TEMP", "VISA Out"=w1428) -> ("error out"=w1419:errorcluster, "ReadValue"=w1433:string, "dup VISA session"=w1425:refnum<visa-resource-name>)  [unwired: 1 out]
            n707 = Format Into String(format string="SENS:AVER %d", error in=w1419, w1423) -> (resulting string=w1424:string, error out=w1418:errorcluster)  [unwired: 1 in]
            n708 = call "PM100D_Write.vi"("error in (no error)"=w1418, "Command"=w1424, "VISA in"=w1425) -> ("error out"=w1417:errorcluster, "VISA out"=w1421:refnum<visa-resource-name>)
            n709 = Fract/Exp String To Number(use system decimal point (T)=FALSE, string=w1433) -> (number=w1431:dbl)  [unwired: 2 in, 1 out]
            n710 = call <vilib>:"Clear Errors.vi"("error in (no error)"=w1417) -> ()  [unwired: 5 in, 2 out]
          }
          frame "Res" {
            (unwired) FALSE
            n711 = call "PM100D_Write.vi"("Command"="SENS:AVER 1", "VISA in"=w1449) -> ("error out"=w1440:errorcluster, "VISA out"=w1448:refnum<visa-resource-name>)  [unwired: 1 in]
            n712 = call "PM100D_Meas.vi"("error in"=w1440, "Timeout"=10 ("Aver"), "ConfPara"="RES", "VISA Out"=w1448) -> ("error out"=w1439:errorcluster, "ReadValue"=w1453:string, "dup VISA session"=w1445:refnum<visa-resource-name>)  [unwired: 1 out]
            n713 = Format Into String(format string="SENS:AVER %d", error in=w1439, w1443) -> (resulting string=w1444:string, error out=w1438:errorcluster)  [unwired: 1 in]
            n714 = Fract/Exp String To Number(use system decimal point (T)=FALSE, string=w1453) -> (number=w1451:dbl)  [unwired: 2 in, 1 out]
            n715 = call "PM100D_Write.vi"("error in (no error)"=w1438, "Command"=w1444, "VISA in"=w1445) -> ("error out"=w1437:errorcluster, "VISA out"=w1441:refnum<visa-resource-name>)
            n716 = call <vilib>:"Clear Errors.vi"("error in (no error)"=w1437) -> ()  [unwired: 5 in, 2 out]
          }
          frame "Min" {
            n717 = Concatenate Strings("%.;%_4" ("format string"), w1459) -> (w1458:string)
          }
        }
        n718 = case shown="\"Off\", Default" w1152 {
          tunnel: ["%d" w1285 w1290 w1322 w1336] -> w1159
          tunnel: ["" "Max:  " "Ratio:  " "D: " ""] -> w1157
          tunnel: [0.0 ("min value") w1286 w1292 w1323 w1338] -> w1154
          tunnel: w1150 -> [_ w1286 w1294 _ _]
          tunnel: w1149 -> [_ _ w1293 _ _]
          tunnel: w1147 -> [_ w1283 _ w1318 _]
          tunnel: w1104 -> [_ _ w1291 w1320 w1340]
          tunnel: w1117 -> [_ _ _ w1325 w1339]
          tunnel: w1115 -> [w1278 w1282 w1288 w1316 w1335]
          tunnel: w1137 -> [_ _ _ _ w1334]
          tunnel: [w1278 w1282 w1288 w1316 w1333] -> w1114
          frame "Off", Default {
            (unwired) FALSE
          }
          frame "Max" {
            n719 = Concatenate Strings("%.;%_4" ("format string"), w1283) -> (w1285:string)
          }
          frame "Ratio" {
            (unwired) FALSE
            n720 = case shown="\"W\", Default" w1291 {
              tunnel: w1294 -> [w1299 w1303 w1307 w1311 w1314]
              tunnel: w1293 -> [w1298 w1302 w1306 w1310 w1315]
              tunnel: [w1297 w1301 w1305 w1309 w1313] -> w1292
              tunnel: [w1296 w1300 w1304 w1308 "%.;%_4fdB" ("format string")] -> w1290
              tunnel: "%.;%_6f:1" ("format string") -> [w1296 w1300 w1304 w1308 _]
              frame "W", Default {
                n721 = Divide(x=w1299, y=w1298) -> (x/y=w1297:dbl)
              }
              frame "V" {
                n722 = Divide(x=w1303, y=w1302) -> (x/y=w1301:dbl)
              }
              frame "J" {
                n723 = Divide(x=w1307, y=w1306) -> (x/y=w1305:dbl)
              }
              frame "A" {
                n724 = Divide(x=w1311, y=w1310) -> (x/y=w1309:dbl)
              }
              frame "dBm" {
                n725 = Subtract(x=w1314, y=w1315) -> (x-y=w1313:dbl)
              }
            }
          }
          frame "Area" {
            (unwired) FALSE
            n726 = local read "AOutcm²"() -> (w1324:dbl)
            n727 = case shown="\"A\"" w1320 {
              tunnel: [w1327 w1328 "pW" ("string") w1330 w1331] -> w1317
              tunnel: w1318 -> [w1327 w1328 _ w1330 w1331]
              frame "W", Default {
              }
              frame "J" {
              }
              frame "dBm" {
              }
              frame "A" {
              }
              frame "V" {
              }
            }
            n728 = Divide(x=w1325, y=w1324) -> (x/y=w1323:dbl)
            n729 = Concatenate Strings("%.;%_4" ("format string"), w1317, "/cm²" ("string")) -> (w1322:string)
          }
          frame "Second" {
            n730 = case shown="\"V\"" w1340 {
              tunnel: w1339 -> [w1345 _ _ _ _]
              tunnel: [w1344 w1350 w1371 w1379 w1387] -> w1338
              tunnel: ["%.;%_6fdBm" ("string") w1349 "%.;%_5pW" ("string") "%.;%_5pW" ("string") "%.;%_5pV" ("string")] -> w1336
              tunnel: w1335 -> [w1342 w1351 w1374 w1382 w1390]
              tunnel: w1334 -> [_ w1348 _ _ _]
              tunnel: [w1342 w1347 w1369 w1377 w1385] -> w1333
              tunnel: [errorcluster {"status"=FALSE, "code"=0, "source"=""} ("error out") w1346 w1368 w1376 w1384] -> w1332
              frame "W", Default {
                n731 = call "lin-log.vi"("W In 2"=w1345) -> ("dBm Out 2"=w1344:dbl)  [unwired: 3 in, 3 out]
              }
              frame "V" {
                n732 = case shown="True" w1348 {
                  tunnel: w1351 -> [w1358 w1366]
                  tunnel: [w1355 w1363] -> w1350
                  tunnel: ["%.;%_5pW" ("string") "%.;%_5pJ" ("string")] -> w1349
                  tunnel: [w1353 w1361] -> w1347
                  tunnel: [w1352 w1360] -> w1346
                  frame False {
                    n733 = call "PM100D_Read.vi"("Command"="MEAS?", "VISA in"=w1358) -> ("error out"=w1352:errorcluster, "ReadValue"=w1356:string, "VISA out"=w1353:refnum<visa-resource-name>)  [unwired: 2 in]
                    n734 = Fract/Exp String To Number(use system decimal point (T)=FALSE, string=w1356) -> (number=w1355:dbl)  [unwired: 2 in, 1 out]
                  }
                  frame True {
                    n735 = call "PM100D_Read.vi"("Command"="MEAS:ENER?", "VISA in"=w1366) -> ("error out"=w1360:errorcluster, "ReadValue"=w1364:string, "VISA out"=w1361:refnum<visa-resource-name>)  [unwired: 2 in]
                    n736 = Fract/Exp String To Number(use system decimal point (T)=FALSE, string=w1364) -> (number=w1363:dbl)  [unwired: 2 in, 1 out]
                  }
                }
              }
              frame "dBm" {
                n737 = call "PM100D_Read.vi"("Command"="MEAS?", "VISA in"=w1374) -> ("error out"=w1368:errorcluster, "ReadValue"=w1372:string, "VISA out"=w1369:refnum<visa-resource-name>)  [unwired: 2 in]
                n738 = Fract/Exp String To Number(use system decimal point (T)=FALSE, string=w1372) -> (number=w1371:dbl)  [unwired: 2 in, 1 out]
              }
              frame "A" {
                n739 = call "PM100D_Read.vi"("Command"="MEAS?", "VISA in"=w1382) -> ("error out"=w1376:errorcluster, "ReadValue"=w1380:string, "VISA out"=w1377:refnum<visa-resource-name>)  [unwired: 2 in]
                n740 = Fract/Exp String To Number(use system decimal point (T)=FALSE, string=w1380) -> (number=w1379:dbl)  [unwired: 2 in, 1 out]
              }
              frame "J" {
                n741 = call "PM100D_Read.vi"("Command"="MEAS:VOLT?", "VISA in"=w1390) -> ("error out"=w1384:errorcluster, "ReadValue"=w1388:string, "VISA out"=w1385:refnum<visa-resource-name>)  [unwired: 2 in]
                n742 = Fract/Exp String To Number(use system decimal point (T)=FALSE, string=w1388) -> (number=w1387:dbl)  [unwired: 2 in, 1 out]
              }
            }
            n743 = call <vilib>:"Clear Errors.vi"("error in (no error)"=w1332) -> ()  [unwired: 5 in, 2 out]
          }
        }
        n744 = case shown="True" w1107 {
          tunnel: w1105 -> [_ w1169]
          frame False {
          }
          frame True {
            n745 = VISA Clear(VISA resource name=w1169) -> (error out=w1167:errorcluster)  [unwired: 1 in, 1 out]
            n746 = call <vilib>:"Clear Errors.vi"("error in (no error)"=w1167) -> ()  [unwired: 5 in, 2 out]
            n747 = local write "Readout"("High") -> ()
          }
        }
        n748 = Format Into String(format string=w1160, initial string=w1158, w1155) -> (resulting string=w1136:string, error out=w1119:errorcluster)  [unwired: 1 in]
        n749 = Format Into String(format string=w1159, initial string=w1157, w1154) -> (resulting string=w1135:string, error out=w1118:errorcluster)  [unwired: 1 in]
        n750 = call <vilib>:"Clear Errors.vi"("error in (no error)"=w1119) -> ()  [unwired: 5 in, 2 out]
        n751 = case shown="True" TRUE {
          tunnel: [w1272 w1274] -> w1145
          tunnel: w1114 -> [_ w1277]
          tunnel: w1104 -> [_ w1275]
          frame False {
            n752 = local read "SlideMulti"() -> (w1272:dbl)
          }
          frame True {
            n753 = call "PM100D_GetRngLbl.vi"("PM100D"=w1277, "MainUnits"=w1275) -> ("String"=w1276:string, "Numeric"=w1274:dbl, "Auto"=w1273:bool)
            n754 = local write "AUTO?"(w1273) -> ()
            n755 = property on="Button1" class="Bool (strict)"("BoolText.Text"=w1276) -> ()  [unwired: 2 in, 2 out]
          }
        }
        n756 = call <vilib>:"Clear Errors.vi"("error in (no error)"=w1118) -> ()  [unwired: 5 in, 2 out]
        n757 = Equal?(x="0", y=w1135) -> (x = y?=w1141:bool)
        n758 = Equal?(x="0", y=w1136) -> (x = y?=w1144:bool)
        n759 = Select(t="", s=w1141, f=w1135) -> (s? t:f=w1131:string)
        n760 = Select(t="", s=w1144, f=w1136) -> (s? t:f=w1130:string)
        n761 = local write "Sub2"(w1131) -> ()
        n762 = local write "Sub1"(w1130) -> ()
        n763 = flat-sequence {
          tunnel: [w1465] -> w1161
          frame #0 {
            n764 = local read "LTM"() -> (w1463:bool)
            n765 = case shown="False" w1463 {
              frame False {
              }
              frame True {
                n766 = local read "PM100D"() -> (w1467:refnum<visa-resource-name>)
                n767 = local read "Interval"() -> (w1466:dbl)
                n768 = Wait (ms)(milliseconds to wait=w1466) -> ()  [unwired: 1 out]
                n769 = call "PM100D_Close.vi"("VISA resource name"=w1467) -> ()  [unwired: 3 in]
              }
            }
            n770 = local write "Button7"(FALSE ("Button7")) -> ()
            n771 = local read "Frame"() -> (w1465:T1)
          }
        }
        n772 = Multiply(x=w1139, y=w1145) -> (x*y=w1156:dbl)
        n773 = local write "Readout"(w1127) -> ()
        n774 = local write "Data"(w1139) -> ()
        n775 = local write "Slide"(w1156) -> ()
      }
      frame "130" {
        n776 = local read "PM100D"() -> (w1470:refnum<visa-resource-name>)
        n777 = call "PM100D_Read.vi"("Command"="MEAS?", "VISA in"=w1470) -> ("error out"=w1469:errorcluster, "ReadValue"=w1480:string)  [unwired: 2 in, 1 out]
        n778 = local read "Unt"() -> (w1475:string)
        n779 = Unbundle By Name(w1469) -> ("status"=w1468:bool)
        n780 = call <vilib>:"Clear Errors.vi"("error in (no error)"=w1469) -> ()  [unwired: 5 in, 2 out]
        n781 = Equal?(x=w1475, y="dBm") -> (x = y?=w1473:bool)
        n782 = Fract/Exp String To Number(use system decimal point (T)=FALSE, string=w1480) -> (number=w1476:dbl)  [unwired: 2 in, 1 out]
        n783 = local read "Samples"() -> (w1478:u32)
        n784 = case shown="True" w1468 {
          tunnel: w1470 -> [_ w1491]
          frame False {
          }
          frame True {
            n785 = VISA Clear(VISA resource name=w1491) -> (error out=w1490:errorcluster)  [unwired: 1 in, 1 out]
            n786 = call <vilib>:"Clear Errors.vi"("error in (no error)"=w1490) -> ()  [unwired: 5 in, 2 out]
          }
        }
        n787 = local read "N"() -> (w1484:u32)
        n788 = case shown="True" w1473 {
          tunnel: w1476 -> [w1492 w1494]
          tunnel: [w1492 w1493] -> w1472
          frame False {
          }
          frame True {
            n789 = Multiply(x=w1494, y=1000.0) -> (x*y=w1496:dbl)
            n790 = Logarithm Base 10(1:w1496) -> (0:w1498:dbl)
            n791 = Multiply(x=10.0, y=w1498) -> (x*y=w1493:dbl)
          }
        }
        n792 = Increment(x=w1484) -> (x+1=w1483:u32)
        n793 = local read "FileRefnum"() -> (w1488:refnum<file>)
        n794 = local read "EMM"() -> (w1485:bool)
        n795 = call "GetDateTime.vi"() -> ("date&time"=w1471:string)
        n796 = local write "N"(w1483) -> ()
        n797 = Number To Decimal String(number=w1483) -> (decimal integer string=w1477:string)  [unwired: 1 in]
        n798 = Equal?(x=w1478, y=w1483) -> (x = y?=w1487:bool)
        n799 = local write "Stat1"(w1477) -> ()
        n800 = case shown="True" w1485 {
          tunnel: [w1513 w1518] -> w1486
          tunnel: w1472 -> [w1512 w1517]
          tunnel: w1471 -> [w1511 w1516]
          tunnel: w1475 -> [w1509 w1515]
          frame True {
            n801 = local read "T"() -> (w1510:dbl)
            n802 = local read "H"() -> (w1508:dbl)
            n803 = Format Into String(format string="\\t%.4e\\t%s\\t%.1f\\t°C\\t%.1f\\tRH\\n", initial string=w1511, w1512, w1509, w1510, w1508) -> (resulting string=w1513:string)  [unwired: 1 in, 1 out]
          }
          frame False {
            n804 = Format Into String(format string="\\t%.4e\\t%s\\n", initial string=w1516, w1517, w1515) -> (resulting string=w1518:string)  [unwired: 1 in, 1 out]
          }
        }
        n805 = Write to Text File(file (use dialog)=w1488, text=w1486) -> (refnum out=w1489:refnum<file>)  [unwired: 2 in, 2 out]
        n806 = case shown="True" w1487 {
          tunnel: w1489 -> [_ w1507]
          tunnel: [w1499 StateMachine."300" ("Frame")] -> w1482
          frame False {
            n807 = local read "Button6"() -> (w1501:bool)
            n808 = Select(t=StateMachine."130" ("Beginning State"), s=w1501, f=StateMachine."300") -> (s? t:f=w1499:T1)
          }
          frame True {
            n809 = Refnum to Path(1:w1507) -> (0:w1506:path)
            n810 = local write "LFP"(w1506) -> ()
            n811 = local write "Button6"(FALSE ("Button6")) -> ()
            n812 = local write "N"(u32 0 ("N")) -> ()
          }
        }
      }
      frame "140" {
        w1541 = 0 ("t")
        w1540 = 2
        # "Energiemessung"
        n813 = local read "MainUnits"() -> (w1566:enum16{"W", "V", "J", "dBm", "A"})
        n814 = local read "PM100D"() -> (w1544:refnum<visa-resource-name>)
        n815 = local read "Digits"() -> (w1565:i32)
        n816 = local read "Button7"() -> (w1547:bool)
        n817 = local read "SensType"() -> (w1553:i32)
        n818 = local read "Sub1"() -> (w1573:enum16{"Off", "Min", "Freq", "Temp", "Res"})
        n819 = local read "Sub2"() -> (w1572:enum16{"Off", "Max", "Ratio", "Area", "Second"})
        n820 = local read "N2"() -> (w1521:u32)
        n821 = local read "AVG"() -> (w1546:u32)
        n822 = local read "EMM"() -> (w1522:bool)
        n823 = Increment(x=w1521) -> (x+1=w1520:u32)
        n824 = local write "N2"(w1520) -> ()
        n825 = Equal?(x=w1553, y=3) -> (x = y?=w1551:bool)
        n826 = case shown="True" w1522 {
          frame False {
          }
          frame True {
            n827 = local read "N2"() -> (w1582:u32)
            n828 = Equal?(x=w1582, y=u32 20) -> (x = y?=w1583:bool)
            n829 = case shown="True" w1583 {
              frame False {
              }
              frame True {
                n830 = local read "PM100D"() -> (w1596:refnum<visa-resource-name>)
                n831 = call "PM100D_Read.vi"("Command"="SENS3:TEMP:DATA?" ("write buffer"), "VISA in"=w1596) -> ("error out"=w1586:errorcluster, "ReadValue"=w1592:string, "VISA out"=w1595:refnum<visa-resource-name>)  [unwired: 2 in]
                n832 = Equal?(x="", y=w1592) -> (x = y?=w1593:bool)
                n833 = case shown="False" w1593 {
                  tunnel: w1592 -> [w1607 _]
                  frame False {
                    n834 = Fract/Exp String To Number(use system decimal point (T)=FALSE, string=w1607) -> (number=w1603:dbl)  [unwired: 2 in, 1 out]
                    n835 = local write "T"(w1603) -> ()
                    n836 = Format Into String(format string="%.;%.1f\\B0C", w1603) -> (resulting string=w1605:string)  [unwired: 2 in, 1 out]
                    n837 = local write "Temp"(w1605) -> ()
                  }
                  frame True {
                  }
                }
                n838 = call "PM100D_Read.vi"("error in (no error)"=w1586, "Command"="SENS2:HUM:DATA?" ("write buffer"), "VISA in"=w1595) -> ("error out"=w1591:errorcluster, "ReadValue"=w1588:string)  [unwired: 1 in, 1 out]
                n839 = call <vilib>:"Clear Errors.vi"("error in (no error)"=w1591) -> ()  [unwired: 5 in, 2 out]
                n840 = Equal?(x=w1588, y="") -> (x = y?=w1589:bool)
                n841 = case shown="False" w1589 {
                  tunnel: w1588 -> [w1599 _]
                  frame False {
                    n842 = Fract/Exp String To Number(use system decimal point (T)=FALSE, string=w1599) -> (number=w1598:dbl)  [unwired: 2 in, 1 out]
                    n843 = Format Into String(format string="%.;%.1f%", w1598) -> (resulting string=w1601:string)  [unwired: 2 in, 1 out]
                    n844 = local write "Hum"(w1601) -> ()
                    n845 = local write "H"(w1598) -> ()
                  }
                  frame True {
                  }
                }
                n846 = local write "N2"(u32 0 ("N2")) -> ()
              }
            }
          }
        }
        n847 = call "PM100D_Read.vi"("Command"="FETC?", "VISA in"=w1544) -> ("error out"=w1543:errorcluster, "ReadValue"=w1527:string, "VISA out"=w1524:refnum<visa-resource-name>)  [unwired: 2 in]
        n848 = call <vilib>:"Clear Errors.vi"("error in (no error)"=w1543) -> ()  [unwired: 5 in, 2 out]
        n849 = Equal?(x=w1527, y="9.91E37\n") -> (x = y?=w1532:bool)
        n850 = Equal?(x=w1527, y="-9.9E37\n") -> (x = y?=w1533:bool)
        n851 = Build Array(w1532, w1533) -> (w1531:bool[])
        n852 = Boolean Array To Number(Boolean array=w1531) -> (number=w1530:u32)
        n853 = case shown="0, Default" w1530 {
          tunnel: [w1615 w1657 w1666] -> w1568
          tunnel: w1566 -> [w1614 w1656 w1665]
          tunnel: w1565 -> [w1613 _ _]
          tunnel: [w1612 w1654 w1663] -> w1563
          tunnel: [w1611 w1654 w1663] -> w1554
          tunnel: [w1610 "High     " "Low     "] -> w1548
          tunnel: w1527 -> [w1609 _ _]
          frame 0, Default {
            n854 = Number To Decimal String(number=w1613) -> (decimal integer string=w1616:string)  [unwired: 1 in]
            n855 = case shown="\"W\", Default" w1614 {
              tunnel: [w1622 w1629 w1636 w1644 w1651] -> w1617
              tunnel: [w1619 w1626 w1633 w1643 w1648] -> w1612
              tunnel: w1616 -> [w1623 w1630 w1637 w1645 w1652]
              tunnel: [w1621 w1628 w1635 w1642 w1650] -> w1615
              tunnel: [w1619 w1626 w1633 w1640 w1648] -> w1611
              tunnel: w1609 -> [w1618 w1625 w1632 w1639 w1647]
              frame "W", Default {
                w1621 = "pW" ("string")
                n856 = Fract/Exp String To Number(use system decimal point (T)=FALSE, string=w1618) -> (number=w1619:dbl)  [unwired: 2 in, 1 out]
                n857 = Concatenate Strings("%.;%_" ("string"), w1623, w1621) -> (w1622:string)
              }
              frame "V" {
                w1628 = "pV" ("string")
                n858 = Fract/Exp String To Number(use system decimal point (T)=FALSE, string=w1625) -> (number=w1626:dbl)  [unwired: 2 in, 1 out]
                n859 = Concatenate Strings("%.;%_" ("string"), w1630, w1628) -> (w1629:string)
              }
              frame "J" {
                w1635 = "pJ" ("string")
                n860 = Fract/Exp String To Number(use system decimal point (T)=FALSE, string=w1632) -> (number=w1633:dbl)  [unwired: 2 in, 1 out]
                n861 = Concatenate Strings("%.;%_" ("string"), w1637, w1635) -> (w1636:string)
              }
              frame "dBm" {
                w1642 = "fdBm" ("string")
                n862 = Fract/Exp String To Number(use system decimal point (T)=FALSE, string=w1639) -> (number=w1640:dbl)  [unwired: 2 in, 1 out]
                n863 = call "lin-log.vi"("W In 2"=w1640) -> ("dBm Out 2"=w1643:dbl)  [unwired: 3 in, 3 out]
                n864 = Concatenate Strings("%.;%_" ("string"), w1645, w1642) -> (w1644:string)
              }
              frame "A" {
                w1650 = "pA" ("string")
                n865 = Fract/Exp String To Number(use system decimal point (T)=FALSE, string=w1647) -> (number=w1648:dbl)  [unwired: 2 in, 1 out]
                n866 = Concatenate Strings("%.;%_" ("string"), w1652, w1650) -> (w1651:string)
              }
            }
            n867 = Format Into String(format string=w1617, w1612) -> (resulting string=w1610:string, error out=w1608:errorcluster)  [unwired: 2 in]
            n868 = call <vilib>:"Clear Errors.vi"("error in (no error)"=w1608) -> ()  [unwired: 5 in, 2 out]
          }
          frame 1 {
            w1654 = 0.0
            n869 = case shown="\"W\", Default" w1656 {
              tunnel: ["W" ("string") "V" ("string") "J" ("string") "A" ("string") "dBm" ("string")] -> w1657
              frame "W", Default {
              }
              frame "V" {
              }
              frame "J" {
              }
              frame "A" {
              }
              frame "dBm" {
              }
            }
          }
          frame 2 {
            w1663 = 0.0
            n870 = case shown="\"dBm\"" w1665 {
              tunnel: ["W" ("string") "V" ("string") "J" ("string") "A" ("string") "dBm" ("string")] -> w1666
              frame "W", Default {
              }
              frame "V" {
              }
              frame "J" {
              }
              frame "A" {
              }
              frame "dBm" {
              }
            }
          }
        }
        n871 = call <vilib>:"Array Max & Min PtByPt.vi"("input data point"=w1563, "sample length"=0, "initialize"=w1547) -> ("max value"=w1570:dbl, "min value"=w1569:dbl)  [unwired: 3 out]
        n872 = case shown="\"Off\", Default" w1573 {
          tunnel: ["%d" "%.;%_6fHz" "%.;%_3f°C" w1827] -> w1580
          tunnel: ["" "f: " "T: " "Min:  "] -> w1578
          tunnel: [0.0 ("min value") w1799 w1819 w1831] -> w1575
          tunnel: w1569 -> [_ _ _ w1831]
          tunnel: w1568 -> [w1781 w1802 w1822 w1828]
          tunnel: [w1781 w1802 w1822 w1828] -> w1567
          tunnel: w1524 -> [w1779 w1797 w1817 w1825]
          tunnel: w1546 -> [_ w1791 w1811 _]
          tunnel: [errorcluster {"status"=FALSE, "code"=0, "source"=""} ("error out") w1785 w1809 errorcluster {"status"=FALSE, "code"=0, "source"=""} ("error out")] -> w1542
          tunnel: [w1779 w1788 w1807 w1825] -> w1523
          frame "Off", Default {
          }
          frame "Freq" {
            n873 = call "PM100D_Write.vi"("Command"="SENS:AVER 1", "VISA in"=w1797) -> ("error out"=w1789:errorcluster, "VISA out"=w1796:refnum<visa-resource-name>)  [unwired: 1 in]
            n874 = call "PM100D_Meas.vi"("error in"=w1789, "Timeout"=500 ("Aver"), "ConfPara"="FREQ", "VISA Out"=w1796) -> ("error out"=w1787:errorcluster, "ReadValue"=w1801:string, "dup VISA session"=w1794:refnum<visa-resource-name>)  [unwired: 1 out]
            n875 = Format Into String(format string="SENS:AVER %d", error in=w1787, w1791) -> (resulting string=w1792:string, error out=w1786:errorcluster)  [unwired: 1 in]
            n876 = call "PM100D_Write.vi"("error in (no error)"=w1786, "Command"=w1792, "VISA in"=w1794) -> ("error out"=w1785:errorcluster, "VISA out"=w1788:refnum<visa-resource-name>)
            n877 = Fract/Exp String To Number(use system decimal point (T)=FALSE, string=w1801) -> (number=w1799:dbl)  [unwired: 2 in, 1 out]
          }
          frame "Temp" {
            n878 = call "PM100D_Write.vi"("Command"="SENS:AVER 1", "VISA in"=w1817) -> ("error out"=w1808:errorcluster, "VISA out"=w1816:refnum<visa-resource-name>)  [unwired: 1 in]
            n879 = call "PM100D_Meas.vi"("error in"=w1808, "Timeout"=10 ("Aver"), "ConfPara"="TEMP", "VISA Out"=w1816) -> ("error out"=w1806:errorcluster, "ReadValue"=w1821:string, "dup VISA session"=w1813:refnum<visa-resource-name>)  [unwired: 1 out]
            n880 = Format Into String(format string="SENS:AVER %d", error in=w1806, w1811) -> (resulting string=w1812:string, error out=w1805:errorcluster)  [unwired: 1 in]
            n881 = call "PM100D_Write.vi"("error in (no error)"=w1805, "Command"=w1812, "VISA in"=w1813) -> ("error out"=w1809:errorcluster, "VISA out"=w1807:refnum<visa-resource-name>)
            n882 = Fract/Exp String To Number(use system decimal point (T)=FALSE, string=w1821) -> (number=w1819:dbl)  [unwired: 2 in, 1 out]
          }
          frame "Min" {
            n883 = Concatenate Strings("%.;%_4" ("format string"), w1828) -> (w1827:string)
          }
        }
        n884 = case shown="\"Second\"" w1572 {
          tunnel: ["%d" w1682 w1686 w1717 w1730] -> w1579
          tunnel: ["" "Max:  " "Ratio:  " "D: " ""] -> w1577
          tunnel: [0.0 ("min value") w1683 w1688 w1718 w1732] -> w1574
          tunnel: w1570 -> [_ w1683 w1690 _ _]
          tunnel: w1569 -> [_ _ w1689 _ _]
          tunnel: w1567 -> [_ w1680 _ w1713 _]
          tunnel: w1566 -> [_ _ w1687 w1715 w1734]
          tunnel: w1554 -> [_ _ _ w1720 w1733]
          tunnel: w1523 -> [_ _ _ _ w1729]
          tunnel: w1551 -> [_ _ _ _ w1728]
          frame "Off", Default {
            (unwired) FALSE
          }
          frame "Max" {
            n885 = Concatenate Strings("%.;%_4" ("format string"), w1680) -> (w1682:string)
          }
          frame "Ratio" {
            (unwired) FALSE
            n886 = case shown="\"W\", Default" w1687 {
              tunnel: w1690 -> [w1695 w1699 w1703 w1707 w1710]
              tunnel: w1689 -> [w1694 w1698 w1702 w1706 w1711]
              tunnel: [w1693 w1697 w1701 w1705 w1709] -> w1688
              tunnel: [w1692 w1696 w1700 w1704 "%.;%_4fdB" ("format string")] -> w1686
              tunnel: "%.;%_6f:1" ("format string") -> [w1692 w1696 w1700 w1704 _]
              frame "W", Default {
                n887 = Divide(x=w1695, y=w1694) -> (x/y=w1693:dbl)
              }
              frame "V" {
                n888 = Divide(x=w1699, y=w1698) -> (x/y=w1697:dbl)
              }
              frame "J" {
                n889 = Divide(x=w1703, y=w1702) -> (x/y=w1701:dbl)
              }
              frame "A" {
                n890 = Divide(x=w1707, y=w1706) -> (x/y=w1705:dbl)
              }
              frame "dBm" {
                n891 = Subtract(x=w1710, y=w1711) -> (x-y=w1709:dbl)
              }
            }
          }
          frame "Area" {
            (unwired) FALSE
            n892 = local read "AOutcm²"() -> (w1719:dbl)
            n893 = case shown="\"A\"" w1715 {
              tunnel: [w1722 w1723 "pW" ("string") w1725 w1726] -> w1712
              tunnel: w1713 -> [w1722 w1723 _ w1725 w1726]
              frame "W", Default {
              }
              frame "J" {
              }
              frame "dBm" {
              }
              frame "A" {
              }
              frame "V" {
              }
            }
            n894 = Divide(x=w1720, y=w1719) -> (x/y=w1718:dbl)
            n895 = Concatenate Strings("%.;%_4" ("format string"), w1712, "/cm²" ("string")) -> (w1717:string)
          }
          frame "Second" {
            n896 = case shown="\"V\"" w1734 {
              tunnel: w1733 -> [w1738 _ _ _ _]
              tunnel: [w1737 w1742 w1760 w1767 w1774] -> w1732
              tunnel: ["%.;%_6fdBm" ("string") w1741 "%.;%_5pW" ("string") "%.;%_5pW" ("string") "%.;%_5pV" ("string")] -> w1730
              tunnel: w1729 -> [_ w1743 w1763 w1770 w1777]
              tunnel: w1728 -> [_ w1740 _ _ _]
              tunnel: [errorcluster {"status"=FALSE, "code"=0, "source"=""} ("error out") w1739 w1758 w1765 w1772] -> w1727
              frame "W", Default {
                n897 = call "lin-log.vi"("W In 2"=w1738) -> ("dBm Out 2"=w1737:dbl)  [unwired: 3 in, 3 out]
              }
              frame "V" {
                n898 = case shown="False" w1740 {
                  tunnel: w1743 -> [w1749 w1756]
                  tunnel: [w1746 w1753] -> w1742
                  tunnel: ["%.;%_5pW" ("string") "%.;%_5pJ" ("string")] -> w1741
                  tunnel: [w1744 w1751] -> w1739
                  frame False {
                    n899 = call "PM100D_Read.vi"("Command"="MEAS?", "VISA in"=w1749) -> ("error out"=w1744:errorcluster, "ReadValue"=w1747:string)  [unwired: 2 in, 1 out]
                    n900 = Fract/Exp String To Number(use system decimal point (T)=FALSE, string=w1747) -> (number=w1746:dbl)  [unwired: 2 in, 1 out]
                  }
                  frame True {
                    n901 = call "PM100D_Read.vi"("Command"="MEAS:ENER?", "VISA in"=w1756) -> ("error out"=w1751:errorcluster, "ReadValue"=w1754:string)  [unwired: 2 in, 1 out]
                    n902 = Fract/Exp String To Number(use system decimal point (T)=FALSE, string=w1754) -> (number=w1753:dbl)  [unwired: 2 in, 1 out]
                  }
                }
              }
              frame "dBm" {
                n903 = call "PM100D_Read.vi"("Command"="MEAS?", "VISA in"=w1763) -> ("error out"=w1758:errorcluster, "ReadValue"=w1761:string)  [unwired: 2 in, 1 out]
                n904 = Fract/Exp String To Number(use system decimal point (T)=FALSE, string=w1761) -> (number=w1760:dbl)  [unwired: 2 in, 1 out]
              }
              frame "A" {
                n905 = call "PM100D_Read.vi"("Command"="MEAS?", "VISA in"=w1770) -> ("error out"=w1765:errorcluster, "ReadValue"=w1768:string)  [unwired: 2 in, 1 out]
                n906 = Fract/Exp String To Number(use system decimal point (T)=FALSE, string=w1768) -> (number=w1767:dbl)  [unwired: 2 in, 1 out]
              }
              frame "J" {
                n907 = call "PM100D_Read.vi"("Command"="MEAS:VOLT?", "VISA in"=w1777) -> ("error out"=w1772:errorcluster, "ReadValue"=w1775:string)  [unwired: 2 in, 1 out]
                n908 = Fract/Exp String To Number(use system decimal point (T)=FALSE, string=w1775) -> (number=w1774:dbl)  [unwired: 2 in, 1 out]
              }
            }
            n909 = call <vilib>:"Clear Errors.vi"("error in (no error)"=w1727) -> ()  [unwired: 5 in, 2 out]
          }
        }
        n910 = Format Into String(format string=w1580, initial string=w1578, w1575) -> (resulting string=w1550:string, error out=w1526:errorcluster)  [unwired: 1 in]
        n911 = call <vilib>:"Clear Errors.vi"("error in (no error)"=w1542) -> ()  [unwired: 5 in, 2 out]
        n912 = Format Into String(format string=w1579, initial string=w1577, w1574) -> (resulting string=w1549:string, error out=w1525:errorcluster)  [unwired: 1 in]
        n913 = local read "SlideMulti"() -> (w1564:dbl)
        n914 = call <vilib>:"Clear Errors.vi"("error in (no error)"=w1526) -> ()  [unwired: 5 in, 2 out]
        n915 = call <vilib>:"Clear Errors.vi"("error in (no error)"=w1525) -> ()  [unwired: 5 in, 2 out]
        n916 = Equal?(x="0", y=w1550) -> (x = y?=w1562:bool)
        n917 = Equal?(x="0", y=w1549) -> (x = y?=w1558:bool)
        n918 = Select(t="", s=w1562, f=w1550) -> (s? t:f=w1561:string)
        n919 = Select(t="", s=w1558, f=w1549) -> (s? t:f=w1556:string)
        n920 = local write "Sub1"(w1561) -> ()
        n921 = local write "Sub2"(w1556) -> ()
        n922 = Multiply(x=w1554, y=w1564) -> (x*y=w1576:dbl)
        n923 = local write "Readout"(w1548) -> ()
        n924 = local read "XScaleFit"() -> (w1539:bool)
        n925 = local read "YScaleFit"() -> (w1538:bool)
        n926 = local read "YScaleRep"() -> (w1537:bool)
        n927 = flat-sequence {
          tunnel: [StateMachine."150" ("Frame")] -> w1581
          frame #0 {
            n928 = local read "LTM"() -> (w1672:bool)
            n929 = case shown="True" w1672 {
              frame False {
              }
              frame True {
                n930 = local read "PM100D"() -> (w1675:refnum<visa-resource-name>)
                n931 = local read "Interval"() -> (w1676:dbl)
                n932 = call "PM100D_Close.vi"("VISA resource name"=w1675) -> ()  [unwired: 3 in]
                n933 = Wait (ms)(milliseconds to wait=w1676) -> ()  [unwired: 1 out]
              }
            }
            n934 = local write "Button7"(FALSE ("Button7")) -> ()
          }
        }
        n935 = local write "Slide"(w1576) -> ()
        n936 = local write "Data"(w1554) -> ()
        n937 = Boolean To (0,1)(Boolean=w1537) -> (0, 1=w1534:i16)
        n938 = Select(t=w1541, s=w1539, f=w1540) -> (s? t:f=w1536:i32)
        n939 = Select(t=w1541, s=w1538, f=w1540) -> (s? t:f=w1535:i32)
        n940 = property on="Chart_E" class="WFChart (strict)"("XScale.ScaleFit"=w1536, "YScale.ScaleFit"=w1535, "YScale.Mapping Mode"=w1534) -> ()  [unwired: 2 in, 2 out]
      }
      frame "150" {
        n941 = local read "Samples"() -> (w1833:u32)
        n942 = local read "Button1"() -> (w1837:bool)
        n943 = local read "Button2"() -> (w1838:bool)
        n944 = local read "Button3"() -> (w1839:bool)
        n945 = local read "Button4"() -> (w1840:bool)
        n946 = local read "Button5"() -> (w1841:bool)
        n947 = local read "Button6"() -> (w1836:bool)
        n948 = local read "N"() -> (w1834:u32)
        n949 = Increment(x=w1834) -> (x+1=w1835:u32)
        n950 = Greater?(x=w1833, y=w1834) -> (0:w1844:bool)
        n951 = local write "N"(w1835) -> ()
        n952 = Compound Arithmetic op=AND(invert w1837, invert w1838, invert w1839, invert w1840, invert w1841, w1836, w1844) -> (w1843:bool)
        n953 = case shown="True" w1843 {
          tunnel: w1833 -> [w1849 w1862]
          tunnel: w1835 -> [w1850 w1861]
          tunnel: [0 w1865] -> w1842
          tunnel: w1836 -> [w1848 _]
          tunnel: [FALSE TRUE] -> w1832
          frame False {
            n954 = Equal?(x=w1848, y=TRUE) -> (x = y?=w1853:bool)
            n955 = Less?(x=w1850, y=w1849) -> (x < y?=w1852:bool)
            n956 = And(x=w1853, y=w1852) -> (x .and. y?=w1851:bool)
            n957 = case shown="True" w1851 {
              frame False {
                n958 = local write "Button6"(FALSE ("Button6")) -> ()
                n959 = local write "N"(i16 0 ("N")) -> ()
              }
              frame True {
                n960 = local read "N"() -> (w1857:u32)
                n961 = Decrement(x=w1857) -> (x-1=w1858:u32)
                n962 = local write "N"(w1858) -> ()
              }
            }
          }
          frame True {
            n963 = local read "MainUnits"() -> (w1895:enum16{"W", "V", "J", "dBm", "A"})
            n964 = case shown="\"W\", Default" w1895 {
              tunnel: ["W" "V" "J" "W" "A"] -> w1874
              tunnel: [w1925 w1929 w1932 w1937 w1941] -> w1879
              tunnel: [FALSE w1929 TRUE FALSE w1941] -> w1878
              tunnel: [w1925 FALSE w1932 w1937 TRUE] -> w1877
              tunnel: ["Power / W" "Energy / V" "Energy / J" "Power / W" ""] -> w1873
              frame "W", Default {
                w1925 = TRUE
              }
              frame "V" {
                w1929 = TRUE
              }
              frame "J" {
                w1932 = FALSE
              }
              frame "dBm" {
                w1937 = TRUE
              }
              frame "A" {
                w1941 = FALSE
              }
            }
            n965 = Equal?(x=i16 1, y=w1861) -> (x = y?=w1896:bool)
            n966 = local read "EMM"() -> (w1860:bool)
            n967 = call "GetDateTime.vi"() -> ("date&time"=w1859:string)
            n968 = local read "Data"() -> (w1876:dbl)
            n969 = local read "Int."() -> (w1875:i32)
            n970 = property on="Chart_E" class="WFChart (strict)"("Visible"=w1878) -> ()  [unwired: 2 in, 2 out]
            n971 = property on="Chart_P" class="WFChart (strict)"("Visible"=w1877) -> ()  [unwired: 2 in, 2 out]
            n972 = case shown="True" w1860 {
              tunnel: w1876 -> [w1907 w1915]
              tunnel: w1874 -> [w1906 w1914]
              tunnel: [w1905 w1913] -> w1871
              tunnel: w1859 -> [w1904 w1912]
              tunnel: [w1903 w1911] -> w1866
              frame False {
                n973 = Format Into String(format string="\\t%.4e\\t%s\\n", initial string=w1904, w1907, w1906) -> (resulting string=w1903:string, error out=w1905:errorcluster)  [unwired: 1 in]
              }
              frame True {
                n974 = local read "H"() -> (w1909:dbl)
                n975 = local read "T"() -> (w1910:dbl)
                n976 = Format Into String(format string="\\t%.4e\\t%s\\t%.1f\\t°C\\t%.1f\\tRH\\n", initial string=w1912, w1915, w1914, w1910, w1909) -> (resulting string=w1911:string, error out=w1913:errorcluster)  [unwired: 1 in]
              }
            }
            n977 = call <vilib>:"Histogram PtByPt.vi"("initialize"=w1896, "sample length"=w1862, "intervals"=w1875, "x"=w1876) -> ("Histogram Graph"=w1901:T2)  [unwired: 4 in, 3 out]
            n978 = call <vilib>:"Array Max & Min PtByPt.vi"("input data point"=w1876, "sample length"=w1862, "initialize"=w1896) -> ("max value"=w1887:dbl, "min value"=w1888:dbl)  [unwired: 3 out]
            n979 = call <vilib>:"Standard Deviation PtByPt.vi"("x"=w1876, "sample length"=w1862, "initialize"=w1896) -> ("standard deviation"=w1894:dbl, "mean"=w1886:dbl)  [unwired: 1 out]
            n980 = call <vilib>:"RMS PtByPt.vi"("initialize"=w1896, "sample length"=w1862, "x"=w1876) -> ("rms value"=w1885:dbl)  [unwired: 1 in, 1 out]
            n981 = Format Into String(format string="%d\\n%.3p%s\\n%.3p%s\\n%.3p%s\\n%.3p%s\\n%.3p%s", error in=w1871, w1861, w1888, w1874, w1887, w1874, w1886, w1874, w1885, w1874, w1894, w1874) -> (resulting string=w1898:string, error out=w1870:errorcluster)  [unwired: 1 in]
            n982 = local read "LogData"() -> (w1900:string)
            n983 = local write "Unit"(w1873) -> ()
            n984 = local write "Chart_E"(w1876) -> ()
            n985 = call "lin-log.vi"("W In 1"=w1885, "W In 2"=w1886, "W In 3"=w1887, "W In 4"=w1888) -> ("dBm Out 1"=w1889:dbl, "dBm Out 2"=w1890:dbl, "dBm Out 3"=w1891:dbl, "dBm Out 4"=w1892:dbl)
            n986 = Format Into String(format string="%.3fdBm\\n%.3fdBm\\n%.3fdBm\\n%.3fdBm", initial string="\n", error in=w1870, w1892, w1891, w1890, w1889) -> (resulting string=w1883:string, error out=w1869:errorcluster)
            n987 = Concatenate Strings(w1866, w1900) -> (w1902:string)
            n988 = local write "Histogram"(w1901) -> ()
            n989 = local read "FileRefnum"() -> (w1867:refnum<file>)
            n990 = local write "Chart_P"(w1876) -> ()
            n991 = local write "Stat1"(w1898) -> ()
            n992 = local write "Stat0"("Count:\nMin:\nMax:\nMean:\nRMS:\nSigma:" ("Stat0")) -> ()
            n993 = local write "LogData"(w1902) -> ()
            n994 = call <vilib>:"Clear Errors.vi"("error in (no error)"=w1869) -> ()  [unwired: 5 in, 2 out]
            n995 = Select(t=w1883, s=w1879, f="") -> (s? t:f=w1882:string)
            n996 = Write to Text File(file (use dialog)=w1867, text=w1866) -> (refnum out=w1864:refnum<file>)  [unwired: 2 in, 2 out]
            n997 = local write "Stat2"(w1882) -> ()
            n998 = Equal?(x=w1862, y=w1861) -> (x = y?=w1863:bool)
            n999 = case shown="True" w1863 {
              tunnel: [2 0] -> w1865
              tunnel: [StateMachine."100" ("Frame") StateMachine."300" ("Frame")] -> w1868
              tunnel: w1864 -> [_ w1920]
              frame False {
              }
              frame True {
                n1000 = Refnum to Path(1:w1920) -> (0:w1919:path)
                n1001 = local write "LFP"(w1919) -> ()
              }
            }
            n1002 = local write "Frame"(w1868) -> ()
          }
        }
        n1003 = flat-sequence {
          tunnel: [w1944] -> w1845
          frame #0 {
            n1004 = local read "Frame"() -> (w1944:T1)
            n1005 = local write "Button7"(FALSE ("Button7")) -> ()
          }
        }
        n1006 = local write "Log"(w1832) -> ()
        n1007 = property on="Button1" class="Bool (strict)"("Disabled"=w1842) -> ()  [unwired: 2 in, 2 out]
        n1008 = property on="Button2" class="Bool (strict)"("Disabled"=w1842) -> ()  [unwired: 2 in, 2 out]
        n1009 = property on="Button3" class="Bool (strict)"("Disabled"=w1842) -> ()  [unwired: 2 in, 2 out]
        n1010 = property on="Button4" class="Bool (strict)"("Disabled"=w1842) -> ()  [unwired: 2 in, 2 out]
        n1011 = property on="Button5" class="Bool (strict)"("Disabled"=w1842) -> ()  [unwired: 2 in, 2 out]
      }
      frame "200" {
        # "Set Measurement Range\n1. Get lowest Amp or Voltage Range\n2. Calculate Current or Voltage Ranges\n3. Get Range Index\n4. Set New Range Index\n5. Get Range in the desired Unit"
        n1012 = flat-sequence {
          frame #0 {
            n1013 = local read "MainUnits"() -> (w1954:enum16{"W", "V", "J", "dBm", "A"})
            n1014 = local read "PM100D"() -> (w1955:refnum<visa-resource-name>)
            n1015 = local read "AUTO?"() -> (w1946:bool)
            n1016 = case shown="\"W\", Default" w1954 {
              tunnel: ["POW" "VOLT" "ENER" "POW" "CURR"] -> w1953
              tunnel: ["W" "V" "J" "W" "A"] -> w1952
              frame "W", Default {
              }
              frame "V" {
              }
              frame "J" {
              }
              frame "dBm" {
              }
              frame "A" {
              }
            }
            n1017 = call "SetRange.vi"("Unit"=w1953, "AUTO"=w1946, "VISA in"=w1955) -> ("AUTO?"=w1950:bool, "RANG_Val"=w1948:dbl, "RANG_lbl"=w1956:string)  [unwired: 5 in, 1 out]
            n1018 = Divide(x=1000.0, y=w1948) -> (x/y=w1947:dbl)
            n1019 = Concatenate Strings("Range " ("string"), w1956, w1952) -> (w1957:string)
            n1020 = property on="Button1" class="Bool (strict)"("BoolText.Text"=w1957) -> ()  [unwired: 2 in, 2 out]
            n1021 = local write "SlideMulti"(w1947) -> ()
            n1022 = local write "AUTO?"(w1950) -> ()
          }
          frame #1 {
            n1023 = local write "Button1"(FALSE ("Button6")) -> ()
            n1024 = local write "Frame"(StateMachine."100" ("Frame")) -> ()
          }
        }
      }
      frame "220" {
        n1025 = flat-sequence {
          frame #0 {
            n1026 = local read "LambdaMin"() -> (w1972:dbl)
            n1027 = local read "LambdaMax"() -> (w1973:dbl)
            n1028 = local read "Lambda"() -> (w1980:dbl)
            n1029 = local read "SensType"() -> (w1979:i32)
            n1030 = local read "Sensor?"() -> (w1974:bool)
            n1031 = call "SetWavelength.vi"("LambdaIn"=w1980, "LambdaMax"=w1973, "LambdaMin"=w1972, "Sensor?"=w1974, "RespIn"=w1980, "Type"=w1979) -> ("LambdaOut"=w1982:dbl, "RespOut"=w1981:dbl)
            n1032 = case shown="True" w1974 {
              tunnel: w1982 -> [w1985 _]
              tunnel: [w1985 w1994] -> w1975
              tunnel: [w1984 w1993] -> w1976
              tunnel: [w1983 w1992] -> w1977
              tunnel: w1979 -> [_ w1995]
              tunnel: w1981 -> [_ w1994]
              frame True {
                n1033 = Format Into String(format string="%dnm", initial string="Wave ", w1985) -> (resulting string=w1984:string)  [unwired: 1 in, 1 out]
                n1034 = Format Into String(format string="%d", initial string="SENS:CORR:WAV " ("Command"), w1985) -> (resulting string=w1983:string)  [unwired: 1 in, 1 out]
              }
              frame False {
                n1035 = case shown="1" w1995 {
                  tunnel: [w2000 "" ("initial string") "" ("initial string") "" ("initial string")] -> w1999
                  tunnel: [w2000 "%.;%_3pA/W" ("format string") "%.;%_3pV/W" ("format string") "%.;%_3pV/J" ("format string")] -> w1998
                  tunnel: [w2000 "SENS:CORR:POW " ("Command") "SENS:CORR:POW:THER " ("Command") "SENS:CORR:ENER " ("Command")] -> w1997
                  tunnel: [w2000 "%.;%.6e" ("format string") "%.;%.6e" ("format string") "%.;%.6e" ("format string")] -> w1996
                  frame 0, Default {
                    w2000 = "" ("format string")
                  }
                  frame 1 {
                  }
                  frame 2 {
                  }
                  frame 3 {
                  }
                }
                n1036 = Format Into String(format string=w1998, initial string=w1999, w1994) -> (resulting string=w1993:string, error out=w1991:errorcluster)  [unwired: 1 in]
                n1037 = Format Into String(format string=w1996, initial string=w1997, error in=w1991, w1994) -> (resulting string=w1992:string, error out=w1990:errorcluster)
                n1038 = call <vilib>:"Clear Errors.vi"("error in (no error)"=w1990) -> ()  [unwired: 5 in, 2 out]
              }
            }
            n1039 = local read "PM100D"() -> (w1978:refnum<visa-resource-name>)
            n1040 = property on="Button2" class="Bool (strict)"("BoolText.Text"=w1976) -> ()  [unwired: 2 in, 2 out]
            n1041 = local write "Lambda"(w1975) -> ()
            n1042 = call "PM100D_Write.vi"("Command"=w1977, "VISA in"=w1978) -> ("error out"=w1971:errorcluster)  [unwired: 1 in, 1 out]
            n1043 = call <vilib>:"Clear Errors.vi"("error in (no error)"=w1971) -> ()  [unwired: 5 in, 2 out]
          }
          frame #1 {
            n1044 = local write "Button2"(FALSE ("Button6")) -> ()
            n1045 = local write "Frame"(StateMachine."100" ("Frame")) -> ()
          }
        }
      }
      frame "240" {
        n1046 = flat-sequence {
          tunnel: [w2050] -> w2016
          tunnel: w2016 -> [w2115]
          tunnel: [w2112] -> w2015
          frame #0 {
            n1047 = local read "PM100D"() -> (w2054:refnum<visa-resource-name>)
            n1048 = local read "Adapter"() -> (w2048:i16)
            n1049 = local read "ACC"() -> (w2046:string)
            n1050 = local read "Digits"() -> (w2065:i32)
            n1051 = local read "SensType"() -> (w2055:i32)
            n1052 = local read "Tau"() -> (w2051:dbl)
            n1053 = local read "AVG"() -> (w2066:u32)
            n1054 = local read "Trig"() -> (w2069:dbl)
            n1055 = local read "Dia"() -> (w2067:dbl)
            n1056 = local read "BW"() -> (w2072:u16)
            n1057 = local read "Tau?"() -> (w2039:bool)
            n1058 = local read "Sensor?"() -> (w2049:bool)
            n1059 = local read "Att"() -> (w2031:dbl)
            n1060 = case shown="\"AUTO\"" w2046 {
              tunnel: ["ON" "ON" "OFF" "OFF" "AUTO" "AUTO"] -> w2045
              frame "ON", Default {
              }
              frame " ON" {
              }
              frame "OFF" {
              }
              frame " OFF" {
              }
              frame ":AUTO ON" {
              }
              frame "AUTO" {
              }
            }
            n1061 = call "MeasCfg.vi"("DigitsIn"=w2065, "TauIn"=w2051, "AvgIn"=w2066, "TrigIn"=w2069, "DiaIn"=w2067, "AttIn"=w2031, "Type"=w2055, "VISA In"=w2054, "Sensor?"=w2049, "Adapter"=w2048, "BWIn"=w2072, "Tau?"=w2039, "ACCIn"=w2045) -> ("Ini"=w2050:bool, "DiaSet"=w2071:dbl, "ACCOut"=w2053:string, "BWOut"=w2037:u16, "AttOut"=w2019:dbl, "DigitsOut"=w2064:i32, "AvgOut"=w2018:i32, "TauIOut"=w2047:dbl, "TrigOut"=w2052:dbl, "DiaOut"=w2070:dbl, "AOutcm²"=w2068:dbl)  [unwired: 4 in]
            n1062 = local write "AOutcm²"(w2068) -> ()
            n1063 = local write "Digits"(w2064) -> ()
            n1064 = local write "ACC"(w2053) -> ()
            n1065 = local write "Tau"(w2047) -> ()
            n1066 = local write "Trig"(w2052) -> ()
            n1067 = local write "BW"(w2037) -> ()
            n1068 = local write "Dia"(w2071) -> ()
            n1069 = case shown="2" w2055 {
              tunnel: w2054 -> [_ w2084 w2098 w2111]
              tunnel: w2053 -> [_ _ w2096 _]
              tunnel: w2052 -> [_ _ _ w2108]
              tunnel: w2047 -> [_ _ w2093 _]
              tunnel: [errorcluster {"status"=FALSE, "code"=0, "source"=""} ("error out") w2083 w2092 w2107] -> w2038
              tunnel: w2039 -> [_ _ w2090 _]
              tunnel: w2037 -> [_ w2082 _ _]
              tunnel: w2018 -> [w2079 w2081 w2088 _]
              tunnel: [w2079 w2081 w2088 1 ("AvgOut")] -> w2017
              frame 0, Default {
              }
              frame 1 {
                n1070 = Format Into String(format string="%d", initial string="INP:FILT ", w2082) -> (resulting string=w2087:string)  [unwired: 1 in, 1 out]
                n1071 = call "PM100D_Write.vi"("Command"=w2087, "VISA in"=w2084) -> ("error out"=w2083:errorcluster)  [unwired: 1 in, 1 out]
              }
              frame 2 {
                n1072 = Format Into String(format string="INP:THER:ACC %s", w2096) -> (resulting string=w2097:string)  [unwired: 2 in, 1 out]
                n1073 = Wait (ms)(milliseconds to wait=u32 30) -> ()  [unwired: 1 out]
                n1074 = call "PM100D_Write.vi"("Command"=w2097, "VISA in"=w2098) -> ("error out"=w2091:errorcluster, "VISA out"=w2094:refnum<visa-resource-name>)  [unwired: 1 in]
                n1075 = case shown="True" w2090 {
                  tunnel: w2094 -> [_ w2105]
                  tunnel: w2093 -> [_ w2104]
                  tunnel: [w2099 w2101] -> w2092
                  tunnel: w2091 -> [w2099 w2100]
                  frame False {
                  }
                  frame True {
                    n1076 = Format Into String(format string="INP:THER:ACC:TAU %.;%f", w2104) -> (resulting string=w2102:string)  [unwired: 2 in, 1 out]
                    n1077 = call "PM100D_Write.vi"("error in (no error)"=w2100, "Command"=w2102, "VISA in"=w2105) -> ("error out"=w2101:errorcluster)  [unwired: 1 out]
                  }
                }
              }
              frame 3 {
                n1078 = Format Into String(format string="SENS:PEAK %.;%f", w2108) -> (resulting string=w2110:string)  [unwired: 2 in, 1 out]
                n1079 = call "PM100D_Write.vi"("Command"=w2110, "VISA in"=w2111) -> ("error out"=w2107:errorcluster)  [unwired: 1 in, 1 out]
              }
            }
            n1080 = Wait (ms)(milliseconds to wait=u32 30) -> ()  [unwired: 1 out]
            n1081 = local write "Att"(w2019) -> ()
            n1082 = call <vilib>:"Clear Errors.vi"("error in (no error)"=w2038) -> ()  [unwired: 5 in, 2 out]
            n1083 = local read "Samples"() -> (w2060:u32)
            n1084 = local read "File?"() -> (w2057:bool)
            n1085 = local read "Interval"() -> (w2058:dbl)
            n1086 = Number To Fractional String(use system decimal point (T)=FALSE, number=w2070) -> (F-format string=w2034:string)  [unwired: 2 in]
            n1087 = local write "AVG"(w2017) -> ()
            n1088 = Number To Fractional String(use system decimal point (T)=FALSE, number=w2019) -> (F-format string=w2021:string)  [unwired: 2 in]
            n1089 = Concatenate Strings("SENS:CORR:BEAM " ("initial string"), w2034) -> (w2035:string)
            n1090 = Format Into String(format string="%d", initial string="SENS:AVER " ("Command"), w2017) -> (resulting string=w2043:string)  [unwired: 1 in, 1 out]
            n1091 = Concatenate Strings("SENS:CORR " ("string"), w2021) -> (w2029:string)
            n1092 = Format Into String(format string="%.;%.2f %s", initial string="a = ", w2019, " dB") -> (resulting string=w2020:string)  [unwired: 1 in, 1 out]
            n1093 = call "PM100D_Write.vi"("Command"=w2043, "VISA in"=w2054) -> ("error out"=w2040:errorcluster, "VISA out"=w2041:refnum<visa-resource-name>)  [unwired: 1 in]
            n1094 = local write "att"(w2020) -> ()
            n1095 = call "PM100D_Write.vi"("error in (no error)"=w2040, "Command"=w2035, "VISA in"=w2041) -> ("error out"=w2026:errorcluster, "VISA out"=w2028:refnum<visa-resource-name>)
            n1096 = call "PM100D_Write.vi"("error in (no error)"=w2026, "Command"=w2029, "VISA in"=w2028) -> ("error out"=w2027:errorcluster)  [unwired: 1 out]
            n1097 = Divide(x=w2058, y=1000.0) -> (x/y=w2062:dbl)
            n1098 = Format Into String(format string="Samples:    %d\\nInterval:      %.2fs\\nAveraging: %d\\nLog to File: %s", initial string="Logging Parameters\n", w2060, w2062, w2017, w2057) -> (resulting string=w2061:string)  [unwired: 1 in, 1 out]
            n1099 = call <vilib>:"Clear Errors.vi"("error in (no error)"=w2027) -> ()  [unwired: 5 in, 2 out]
            n1100 = local write "LogCfg"(w2061) -> ()
          }
          frame #1 {
            w2113 = StateMachine."100" ("f")
            n1101 = Select(t=StateMachine."Load Settings" ("Frame"), s=w2115, f=w2113) -> (s? t:f=w2112:T1)
            n1102 = local write "Frame"(w2113) -> ()
            n1103 = local write "Button3"(FALSE ("Button6")) -> ()
          }
        }
      }
      frame "260" {
        n1104 = flat-sequence {
          frame #0 {
            n1105 = local read "MainUnits"() -> (w2120:enum16{"W", "V", "J", "dBm", "A"})
            n1106 = local read "SensType"() -> (w2125:i32)
            n1107 = local read "Temp"() -> (w2118:bool)
            n1108 = local read "Sub1"() -> (w2121:enum16{"Off", "Min", "Freq", "Temp", "Res"})
            n1109 = local read "Sub2"() -> (w2122:enum16{"Off", "Max", "Ratio", "Area", "Second"})
            n1110 = call "SetUnits.vi"("Temp"=w2118, "SensType"=w2125, "Sub1In"=w2121, "Sub2In"=w2122, "MainUnitsIn"=w2120) -> ("Sub1Out"=w2119:enum16{"Off", "Min", "Freq", "Temp", "Res"}, "Sub2Out"=w2124:u16, "MainUnitsOut"=w2123:enum16{"W", "V", "J", "dBm", "A"})
            n1111 = local write "MainUnits"(w2123) -> ()
            n1112 = local write "Sub1"(w2119) -> ()
            n1113 = local write "Sub2"(w2124) -> ()
          }
          frame #1 {
            n1114 = local write "Button4"(FALSE ("Button6")) -> ()
            n1115 = local write "Frame"(StateMachine."100" ("Frame")) -> ()
          }
        }
      }
      frame "280" {
        n1116 = flat-sequence {
          frame #0 {
            w2157 = 1000 ("y")
            n1117 = local read "Samples"() -> (w2158:u32)
            n1118 = local read "Header"() -> (w2140:string)
            n1119 = local read "SensType"() -> (w2148:i32)
            n1120 = local read "AVG"() -> (w2160:u32)
            n1121 = local read "File?"() -> (w2159:bool)
            n1122 = local read "Interval"() -> (w2154:dbl)
            n1123 = local read "FastIn"() -> (w2136:bool)
            n1124 = Divide(x=w2154, y=w2157) -> (x/y=w2155:dbl)
            n1125 = call "LogCfg.vi"("SensType"=w2148, "FastIn"=w2136, "FileIn"=w2159, "AveragingIn"=w2160, "IntervalIn"=w2155, "SamplesIn"=w2158) -> ("FileOut"=w2144:bool, "AveragingOut"=w2149:i32, "IntervalOut"=w2156:dbl, "SamplesOut"=w2162:i32, "FastOut"=w2133:bool, "FileRefnum"=w2141:refnum<file>)
            n1126 = Refnum to Path(1:w2141) -> (0:w2147:path)
            n1127 = Concatenate Strings(w2140, "\r\n") -> (w2139:string)
            n1128 = local write "FastOut"(w2133) -> ()
            n1129 = local write "FastIn"(w2133) -> ()
            n1130 = Strip Path(path=w2147) -> (name=w2146:string)  [unwired: 1 out]
            n1131 = Write to Text File(file (use dialog)=w2141, text=w2139) -> (refnum out=w2134:refnum<file>, cancelled=w2135:bool, error out=w2137:errorcluster)  [unwired: 2 in]
            n1132 = Multiply(x=w2156, y=w2157) -> (x*y=w2165:dbl)
            n1133 = case shown="False" w2135 {
              tunnel: w2137 -> [_ w2168]
              tunnel: w2134 -> [w2167 _]
              frame False {
                n1134 = local write "FileRefnum"(w2167) -> ()
                n1135 = Refnum to Path(1:w2167) -> (0:w2166:path)
                n1136 = local write "LFP"(w2166) -> ()
              }
              frame True {
                n1137 = call <vilib>:"Clear Errors.vi"("error in (no error)"=w2168) -> ()  [unwired: 5 in, 2 out]
              }
            }
            n1138 = local write "Samples"(w2162) -> ()
            n1139 = local write "Interval"(w2165) -> ()
            n1140 = local read "PM100D"() -> (w2150:refnum<visa-resource-name>)
            n1141 = local write "File?"(w2144) -> ()
            n1142 = local write "AVG"(w2149) -> ()
            n1143 = Divide(x=w2165, y=1000.0) -> (x/y=w2129:dbl)
            n1144 = Format Into String(format string="%d", initial string="SENS:AVER " ("Command"), w2149) -> (resulting string=w2152:string)  [unwired: 1 in, 1 out]
            n1145 = Select(t=0.0, s=w2133, f=w2129) -> (s? t:f=w2130:dbl)
            n1146 = call "PM100D_Write.vi"("Command"=w2152, "VISA in"=w2150) -> ("error out"=w2142:errorcluster)  [unwired: 1 in, 1 out]
            n1147 = Select(t=w2146, s=w2144, f="") -> (s? t:f=w2145:string)
            n1148 = call <vilib>:"Clear Errors.vi"("error in (no error)"=w2142) -> ()  [unwired: 5 in, 2 out]
            n1149 = Format Into String(format string="Samples:    %d\\nInterval:      %.;%.1fs\\nAveraging: %d\\nLog to File: %s\\n%s", initial string="Logging Parameters\n", w2162, w2130, w2149, w2144, w2145) -> (resulting string=w2164:string)  [unwired: 1 in, 1 out]
            n1150 = local write "LogCfg"(w2164) -> ()
          }
          frame #1 {
            n1151 = local write "Button5"(FALSE ("Button6")) -> ()
            n1152 = local write "Frame"(StateMachine."100" ("Frame")) -> ()
          }
        }
      }
      frame "300" {
        n1153 = flat-sequence {
          frame #0 {
            n1154 = local read "LFP"() -> (w2172:path)
            n1155 = Read from Text File(file (use dialog)=w2172, count=-1) -> (text=w2174:string, cancelled=w2175:bool, error out=w2176:errorcluster)  [unwired: 2 in, 1 out]
            n1156 = case shown="False" w2175 {
              tunnel: w2174 -> [w2178 _]
              tunnel: w2176 -> [_ w2256]
              frame False {
                n1157 = flat-sequence {
                  tunnel: w2178 -> [w2181]
                  tunnel: [w2181] -> w2177
                  tunnel: w2177 -> [w2194]
                  frame #0 {
                    n1158 = local write "Histogram"(T4 {"X Values"=[], "Histogram: h(x)"=[]} ("Histogram Graph")) -> ()
                    n1159 = property on="Chart_P" class="WFChart (strict)"("History Data"=dbl[] []) -> ()  [unwired: 2 in, 2 out]
                  }
                  frame #1 {
                    n1160 = local write "LogData"(w2194) -> ()
                    n1161 = Spreadsheet String To Array(format string="%s", spreadsheet string=w2194, array type (2D Dbl)="") -> (array=w2191:string[][])  [unwired: 1 in]
                    n1162 = Array Subset(array=w2191, index (row)=1 ("index"), index (col)=0 ("index"), length (col)=1 ("length")) -> (w2187:string[][])  [unwired: 1 in]
                    n1163 = Index Array(array=w2187, index (col)=0 ("disabled index (col)")) -> (element=w2185:string[])  [unwired: 1 in]
                    n1164 = Array Subset(array=w2191, index (row)=1 ("index"), index (col)=1 ("index"), length (col)=1 ("length")) -> (w2192:string[][])  [unwired: 1 in]
                    n1165 = Array Subset(array=w2191, index (row)=1 ("index"), index (col)=2 ("index"), length (col)=1 ("length")) -> (w2197:string[][])  [unwired: 1 in]
                    n1166 = local read "Int."() -> (w2195:i32)
                    n1167 = Index Array(array=w2192, index (col)=0 ("disabled index (col)")) -> (element=w2205:string[])  [unwired: 1 in]
                    n1168 = Index Array(array=w2197, index (col)=0 ("disabled index (col)")) -> (element=w2196:string[])  [unwired: 1 in]
                    n1169 = Fract/Exp String To Number(string=w2205, default (0 dbl)=0.0 ("default (0 DBL)")) -> (number=w2186:dbl[])  [unwired: 2 in, 1 out]
                    n1170 = Array Size(array=w2186) -> (size(s)=w2203:i32)
                    n1171 = call <vilib>:"Histogram.vi"("intervals"=w2195, "X"=w2186) -> ("Histogram Graph"=w2202:T2)  [unwired: 6 in, 3 out]
                    n1172 = local write "Histogram"(w2202) -> ()
                    n1173 = for {
                      N: w2203 -> [w2219]
                      tunnel: w2186 -> [w2215] mode=indexing
                      tunnel: w2196 -> [w2247] mode=indexing
                      tunnel: w2185 -> [w2220] mode=indexing
                      tunnel: [w2230] -> w2184 mode=indexing
                      tunnel: [w2215] -> w2183 mode=indexing
                      i -> [w2217]
                      w2229 = " " ("delimiter (Tab)")
                      n1174 = local write "Chart_P"(w2215) -> ()
                      n1175 = local write "Chart_E"(w2215) -> ()
                      n1176 = Equal?(x=0, y=w2217) -> (x = y?=w2252:bool)
                      n1177 = call <vilib>:"Array Max & Min PtByPt.vi"("input data point"=w2215, "sample length"=w2219, "initialize"=w2252) -> ("max value"=w2236:dbl, "min value"=w2237:dbl)  [unwired: 3 out]
                      n1178 = call <vilib>:"Standard Deviation PtByPt.vi"("x"=w2215, "sample length"=w2219, "initialize"=w2252) -> ("standard deviation"=w2248:dbl, "mean"=w2235:dbl)  [unwired: 1 out]
                      n1179 = call <vilib>:"RMS PtByPt.vi"("initialize"=w2252, "sample length"=w2219, "x"=w2215) -> ("rms value"=w2234:dbl)  [unwired: 1 in, 1 out]
                      n1180 = local read "SensType"() -> (w2213:i32)
                      n1181 = Increment(x=w2217) -> (x+1=w2216:i32)
                      n1182 = Equal?(x=w2219, y=w2216) -> (x = y?=w2218:bool)
                      n1183 = Equal?(x=w2247, y="W") -> (x = y?=w2241:bool)
                      n1184 = Spreadsheet String To Array(delimiter (Tab)=w2229, format string="%s", spreadsheet string=w2220, array type (2D Dbl)=string[] []) -> (array=w2224:string[])
                      n1185 = Format Into String(format string="%d\\n%.3p%s\\n%.3p%s\\n%.3p%s\\n%.3p%s\\n%.3p%s", w2219, w2237, w2247, w2236, w2247, w2235, w2247, w2234, w2247, w2248, w2247) -> (resulting string=w2249:string)  [unwired: 2 in, 1 out]
                      n1186 = Equal?(x=w2213, y=3) -> (x = y?=w2212:bool)
                      n1187 = Index Array(array=w2224, index #1=1 ("index"), index #2=0 ("index")) -> (element #1=w2228:string, element #2=w2227:string)
                      n1188 = case shown="False" w2212 {
                        tunnel: w2218 -> [w2254 _]
                        frame False {
                          n1189 = Not(x=w2254) -> (.not. x?=w2255:bool)
                          n1190 = property on="Chart_P" class="WFChart (strict)"("Visible"=w2255) -> ()  [unwired: 2 in, 2 out]
                          n1191 = property on="YT" class="XYGraph (strict)"("Visible"=w2254) -> ()  [unwired: 2 in, 2 out]
                        }
                        frame True {
                        }
                      }
                      n1192 = call "lin-log.vi"("W In 1"=w2234, "W In 2"=w2235, "W In 3"=w2236, "W In 4"=w2237) -> ("dBm Out 1"=w2239:dbl, "dBm Out 2"=w2244:dbl, "dBm Out 3"=w2243:dbl, "dBm Out 4"=w2242:dbl)
                      n1193 = local write "Stat0"("Count:\nMin:\nMax:\nMean:\nRMS:\nSigma:" ("Stat0")) -> ()
                      n1194 = Concatenate Strings(w2228, w2229, w2227) -> (w2221:string)
                      n1195 = local write "Stat1"(w2249) -> ()
                      n1196 = Format Into String(format string="%.3fdBm\\n%.3fdBm\\n%.3fdBm\\n%.3fdBm", initial string="\n", w2242, w2243, w2244, w2239) -> (resulting string=w2232:string)  [unwired: 1 in, 1 out]
                      n1197 = Select(t=w2232, s=w2241, f="") -> (s? t:f=w2233:string)
                      n1198 = Scan From String(input string=w2221, default 1=timestamp(0 s since 1904-01-01)) -> (output 1=w2230:timestamp)  [unwired: 3 in, 3 out]
                      n1199 = local write "Stat2"(w2233) -> ()
                    }
                    n1200 = Bundle(w2184, w2183) -> (w2182:cluster{timestamp[], dbl[]})  [unwired: 1 in]
                    n1201 = local write "YT"(w2182) -> ()
                  }
                }
              }
              frame True {
                n1202 = call <vilib>:"Clear Errors.vi"("error in (no error)"=w2256) -> ()  [unwired: 5 in, 2 out]
              }
            }
          }
          frame #1 {
            n1203 = local write "Imp"(FALSE ("Imp")) -> ()
            n1204 = local write "Frame"(StateMachine."100" ("Frame")) -> ()
          }
        }
      }
      frame "Stop" {
        n1205 = flat-sequence {
          frame #0 {
            w2260 = T21 2 items=["Deassert REN", "Assert REN", "Go To Local; Deassert REN ", "Assert REN; Address Device", "Local Lockout (Addressed Devices)", "Local Lockout (This Device)", "Go To Local"] ("Mode")
            n1206 = local read "PM100D"() -> (w2262:refnum<visa-resource-name>)
            n1207 = disable-structure shown="Enabled" {
              frame Enabled {
                n1208 = local write "Frame"(StateMachine."Initialize" ("Frame")) -> ()
              }
              frame Disabled {
              }
            }
            n1209 = local write "Button8"(FALSE ("Button8")) -> ()
            n1210 = call "PM100D_Close.vi"("Mode"=w2260, "VISA resource name"=w2262) -> ()  [unwired: 2 in]
          }
          frame #1 {
            n1211 = Quit LabVIEW(quit? (T)=TRUE) -> ()
          }
        }
      }
    }
    n1212 = local read "Stop"() -> (w520:bool)
  }
  "Stop" <- FALSE ("Stop")
